vi "信号光谱9-Au-卍-ver1.vi"() -> ()   [LabVIEW 2018]
uses:
  <vilib>/Utility/NIReport.llb/Report Type.ctl
  <vilib>/Utility/file.llb/Write Delimited Spreadsheet (DBL).vi
  <vilib>/Instr/_visa.llb/VISA Configure Serial Port (Instr).vi
  <vilib>/addons/_office/excel.llb/Excel Get Data ([str]).vi
  <vilib>/Utility/NIReport.llb/NI_report.lvclass
  <vilib>/Analysis/NI_AALBase.lvlib
  <vilib>/ptbypt/NI_PtbyPt.lvlib
  <vilib>/Utility/NIReport.llb/NI_ReportGenerationCore.lvlib
  <vilib>/addons/_office/NI_ReportGenerationToolkit.lvlib
  <vilib>/Utility/NIReport.llb/Excel/NI_Excel.lvclass
panel:
  in  "num":i32=1
  in  "角度判断下限":dbl=1.0 format="%#_13g"
  in  "角度判断上限":dbl=4.0 format="%#_13g"
  out "原始峰值":dbl
  out "拟合峰值":dbl
  in  "角度倍乘系数":dbl=1.5
  out "结果展示":dbl[][](array[numeric])=[[37.33100777239877, 2672.955043835526, 29.54153292599307, 222755.0, 50.0], [37.36593979472361, 2672.656498058864, 30.113284142729572, 222833.0, 50.0], [38.96986225690859, 2673.3337152325566, 33.38805102415213, 222910.0, 75.0], [37.39946104045098, 2676.4005085744548, 31.215565446104666, 222948.0, 47.0], [35.862209164247574, 2671.7826876859012, 30.355582265151796, 223028.0, 47.0]]
  out "Δw2>C":bool=TRUE
  out "Δw1>C":bool=TRUE
  out "θi":dbl
  in  "w0":dbl format="%#_13g"
  in  "C=w-w0":dbl=180.0 format="%#_13g"
  in  "上升下降沿/s":dbl format="%.2p"
  in  "延时/s":dbl format="%.2p"
  in  "占空比/%":dbl=3.0 format="%.2p"
  in  "高电平/V":dbl=4.0 format="%.2p"
  in  "频率/Hz":dbl=6000.0 format="%.3p"
  in  "低电平/V":dbl min=0.0 max=5.0 format="%.2p"
  in  "Enable":bool
  in  "上升下降沿":i32(ring)=1 items=["上升沿", "下降沿"]
  in  "输出信号波形":u16(ring) items=["Pulse"]
  out "Output":bool
  in  "VISA 信号发生器":refnum<visa-resource-name>="USB0::0x1AB1::0x0641::DG4E192200870::INSTR"
  out "Output 2":bool
  in  "Enable 2":bool
  in  "上升下降沿/s 2":dbl format="%.2p"
  in  "延时/s 2":dbl format="%.2p"
  in  "占空比/% 2":dbl=3.0 format="%.2p"
  in  "高电平/V 2":dbl=0.002 format="%.2p"
  in  "频率/Hz 2":dbl=6000.0 format="%.3p"
  in  "低电平/V 2":dbl min=0.0 max=5.0 format="%.2p"
  in  "上升下降沿 2":i32(ring)=1 items=["上升沿", "下降沿"]
  in  "输出信号波形 2":u16(ring) items=["Pulse"]
  in  "终止测量":bool
  in  "测量次数":i32=1
  out "best fit":cluster{"Y":dbl[], "Y":dbl[]}[](graph)
  in  "拟合终点":i32=850
  in  "拟合起点":i32=200
  out "angle":dbl
  out "图片地址":string
  in  "开光时间/ms":u32=50
  out "最终存储路径 2":path
  out "照明光error out":errorcluster
  in  "照明光":bool
  in  "stop bits (10: 1 bit)":u16(ring)=10 items=["1.0"=10, "1.5"=15, "2.0"=20]
  in  "parity (0:none)":enum16{"None", "Odd", "Even", "Mark", "Space"}(ring)
  in  "data bits (8)":u16=8 min=5 max=8 step=1
  in  "baud rate":u32=9600 caption="baud rate (115200)" min=9600 max=115200
  in  "照明光VISA":refnum<visa-resource-name>="COM6"
  out "正在测量":bool
  in  "滤波阈值":dbl=3000.0 format="%#_13g"
  out "范围内？":bool[](array[boolean])
  out "w":dbl
  out "xc":dbl
  out "拟合参数":dbl[](array[numeric])
  out "最终存储路径":path
  in  "停止程序":bool
  out "configure error out":errorcluster
  in  "设置参数":bool
  out "output control error  4":errorcluster
  in  "低电平持续输出":bool
  out "output control error  5":errorcluster
  out "output control error":errorcluster
  in  "开始测量":bool
  in  "channel输出口":i32(ring) items=["Channel 1", "Channel 2"]
  out "output control error":errorcluster
  out "Spectrum":cluster{"Y":dbl[], "Y":dbl[]}[](graph)
  out "波长范围":dbl[](array[numeric])
  in  "?":enum32{"IHR 550", "CCD"}(tab)
  in  "Move To\nTarget Positions":bool
  out "Current UniqueID":string="Mono4"
  in  "Mono ID":string(combo)="Mono1"
  in  "Connect":bool
  out "Initialized JY":bool=TRUE
  in  "Force\nInitialization":bool
  in  "Target Grating":string(combo)="2"
  out "Current Description":string="1" caption="Description"
  out "Grating Index":i32=1
  out "Current Grating":dbl=1200.0
  out "Units":string="nm"
  out "Current WL":dbl=897.9988
  out "Exit Mirror\nPosition":i32(ring)=2 items=["EntranceMirror", "ExitMirror", "Front", "Side"]
  out "Entrance Mirror\nPosition":i32(ring)=2 items=["EntranceMirror", "ExitMirror", "Front", "Side"]
  out "Units 2":string="mm"
  out "Front Entrance":dbl
  in  "Target WL":dbl=516.0
  in  "Exit Mirror":u16(ring)=3 caption="Target Position Exit Mirror" items=["Front"=2, "Side"=3]
  in  "Entrance Mirror":u16(ring)=2 caption="Target Position\nEntrance Mirror" items=["Front"=2, "Side"=3]
  in  "Target\nFront Entrance":dbl=1.0
  in  "Commande tab":T1(tab)
  in  "Area Number to Display":i32
  in  "Reformat":bool
  in  "GAIN":u16(ring)=2 caption="Device Name" items=["High Light", "Best Dynamic Range", "High Sensitivity"]
  in  "ADC":u16(ring) caption="Device Name" items=["20 kHz       ", " 1 MHz       ", " 1 MHz Ultra "]
  in  "Number of Areas :":u16=1 min=1 step=1
  in  "Integration time (ms) :":i16=1000
  out "Uniques ID":u16(ring) items=["CCD1", "CCD2"]
  in  "Device Name":u16(ring) items=["Synapse CCD (Lateral)", "Synapse_IGA (Axial)"]
  in  "Signal type :":enum16{"TTL Rising Edge", "TTL Falling Edge"}(ring)=enum."TTL Falling Edge"
  in  "Trigger Type :":u16(ring) items=["On Start"=1, "Per Acquisition"=2]
  in  "trigSigTypeString":string
  in  "trigEventString":string
  in  "Enable InputTriggers :":bool
  in  "Number of Cleans":i32=1
  in  "MultiAcqShutterMode":i32(ring)=3 items=["Open For All Spectra"=1, "Open for Each Spectrum"=3]
  in  "Accumulations:":u16=10 min=1 step=1
  in  "Multi Accumulation mode:":bool
  out "Y Pixels:":i32=256
  out "DataSize":i32=1024
  out "X Pixels:":i32=1024
  out "Firmware\nVersion":string="V1.20 CCD_4000"
  out "initialized ?":bool=TRUE
  in  "Continuous":bool
  in  "CCD Busy":bool
  out "indicator":string="Ready !"
  in  "initialize":bool
  in  "ShutterOpen":bool=TRUE caption="Shutter enable"
  in  "Acquire":bool
  in  "Temperature":bool
  in  "Setup":bool
  out "Acq Time(ms)":u32=3401
  in  "Save Backlight":bool
  in  "cut backlight":bool
  out "backlight":bool=TRUE
  in  "是否拟合":bool
  in  "是否保存":bool
  in  "Close":bool=TRUE
  out "JYCCDLib.IJYCCDReqd":refnum<k7>
  out "areas :":i32[][](array[numeric])=[[1], [1], [1], [1024], [256], [1], [256]]
  in  "Constante de condition\n(Voir l'aide contextuelle)":bool
  out "temp graph":dbl(graph)=-134.538067
  out "ADC Number":i32[](array[numeric])=[0, 1, 2, 3, 4]
  out "Gain Number":i32[](array[numeric])=[10, 11, 12, 13, 8, 2]
  out "trigAddress":i32
  out "Data":i32[][](graph)
  out "error out":errorcluster
  out "Gratings":dbl[](array[numeric])=[1200.0, 300.0]
  out "Backlight":i32[][](graph)
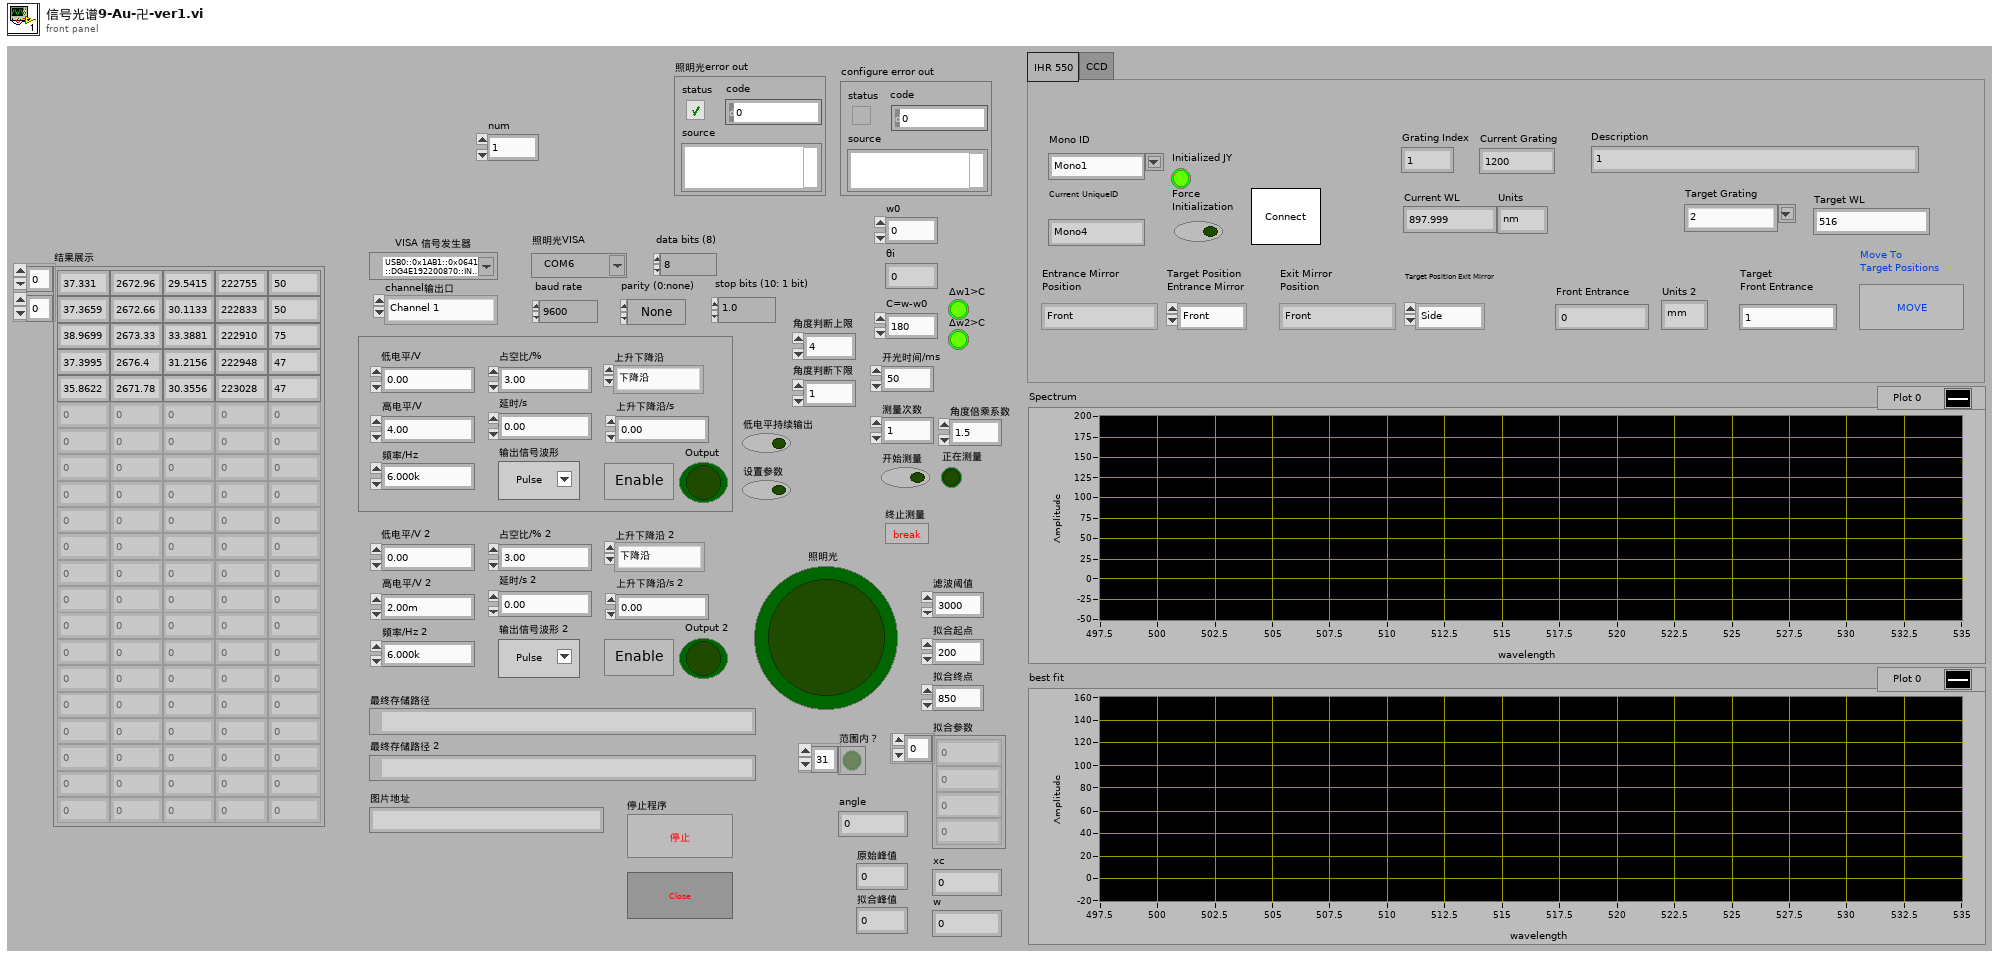
[diagram p1: front panel]
types:
  T1 = enum32{"Settings", "Trigger In", "Multi-Accu.", "Infos"}
  T2 = enum8{"Enabled", "Disabled", "Disabled and Grayed Out"}
  T3 = enum16{"maximized", "minimized", "normal", "no change"}
  T4 = typedef "NI_ReportGenerationCore.lvlib/Report Type.ctl" = enum16{"HTML", "Word", "Excel"}
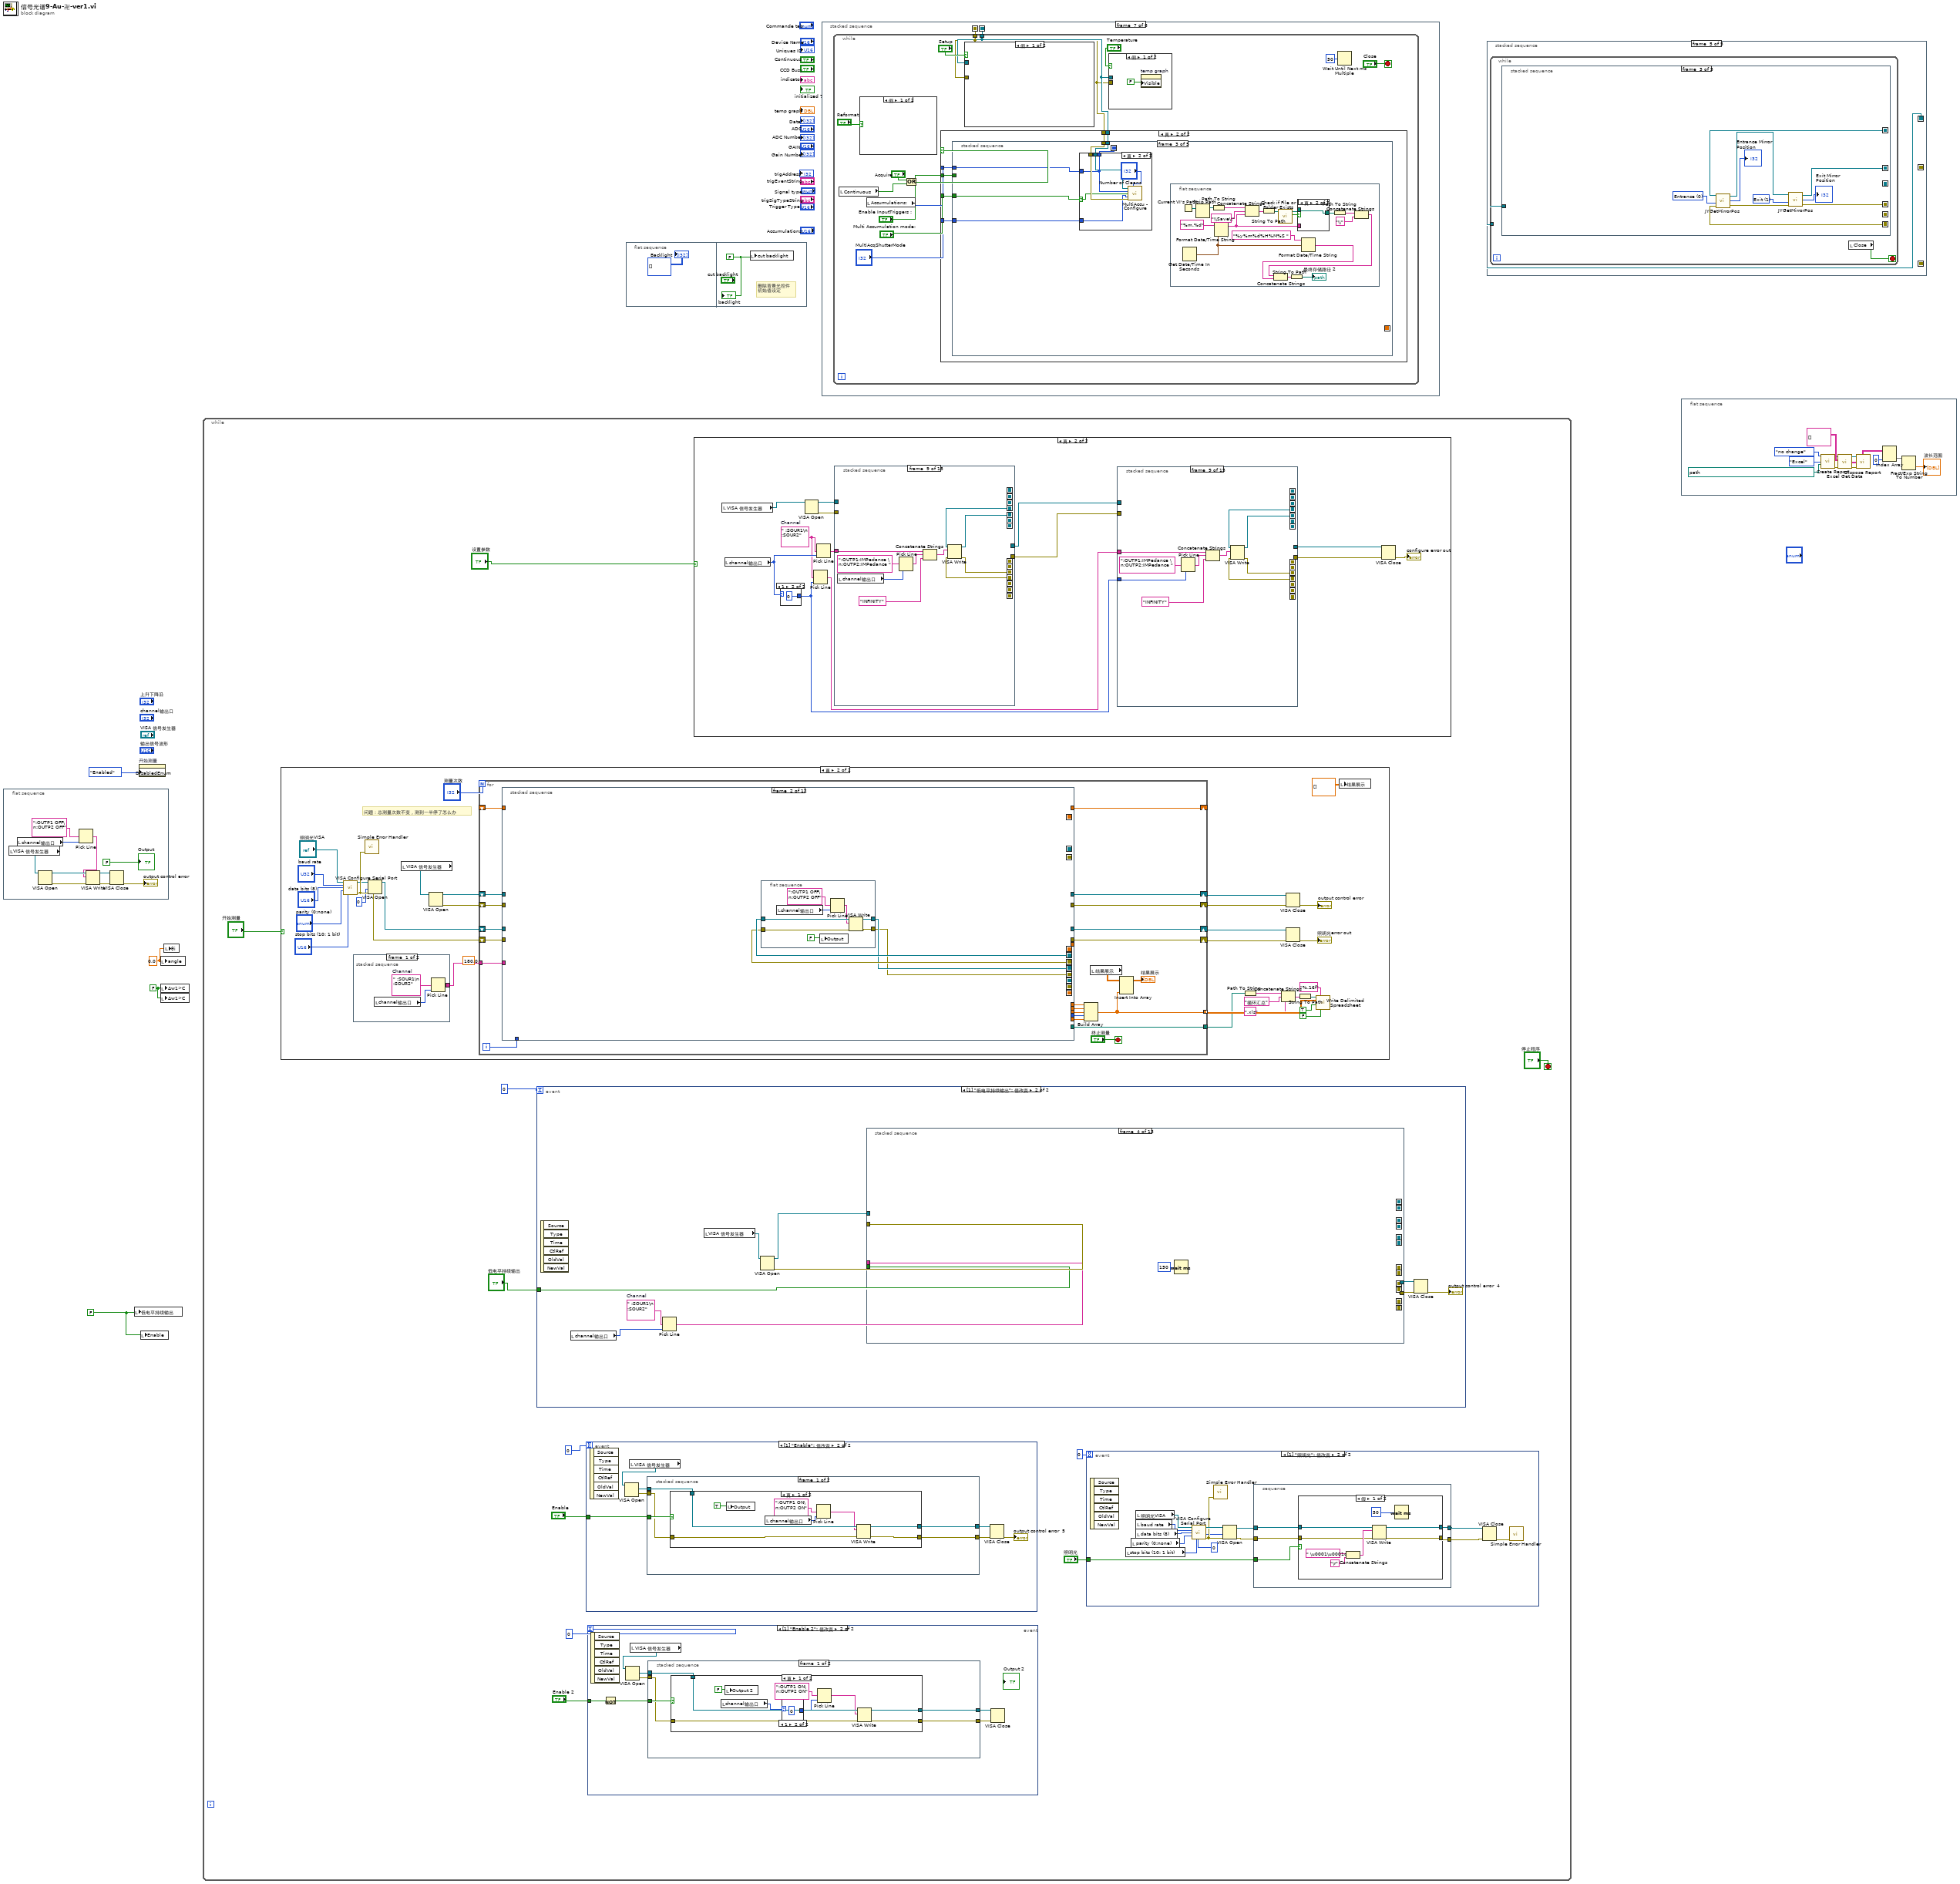
[diagram p0: block diagram]
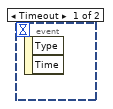
[diagram p2: hidden frame]
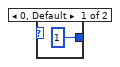
[diagram p3: hidden frame]
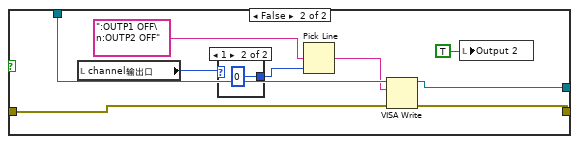
[diagram p4: hidden frame]
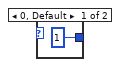
[diagram p5: hidden frame]
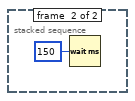
[diagram p6: hidden frame]
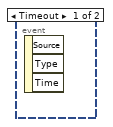
[diagram p7: hidden frame]
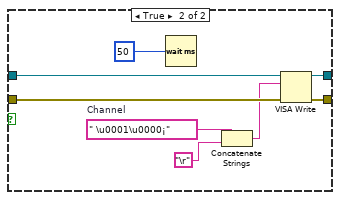
[diagram p8: hidden frame]
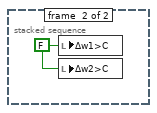
[diagram p10: hidden frame]
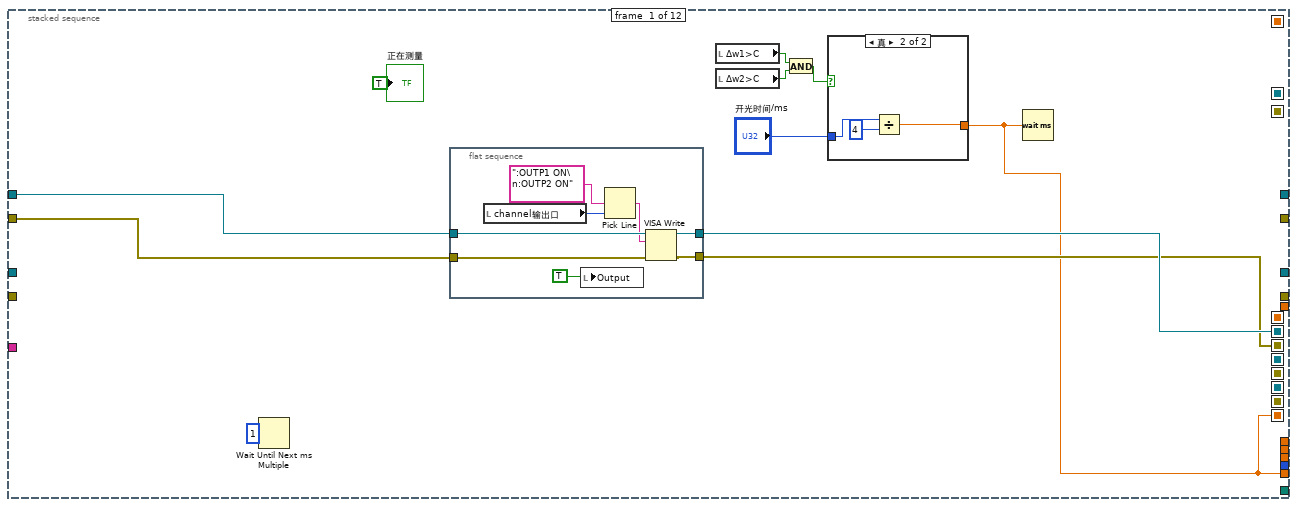
[diagram p11: hidden frame]
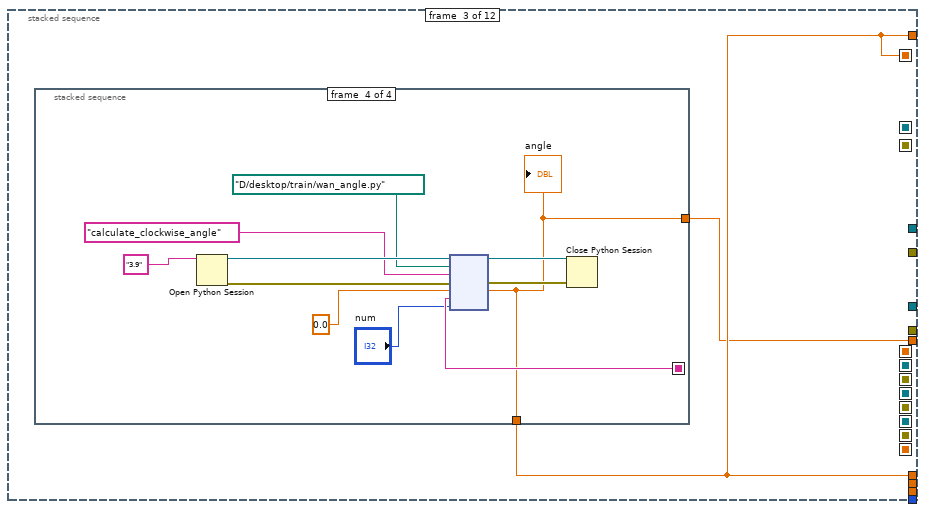
[diagram p13: hidden frame]
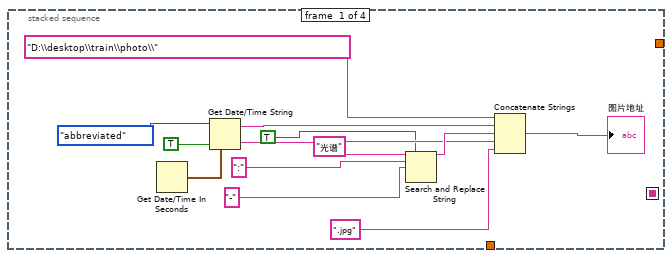
[diagram p14: hidden frame]
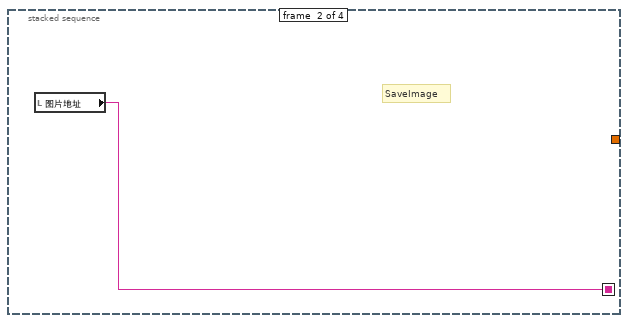
[diagram p15: hidden frame]
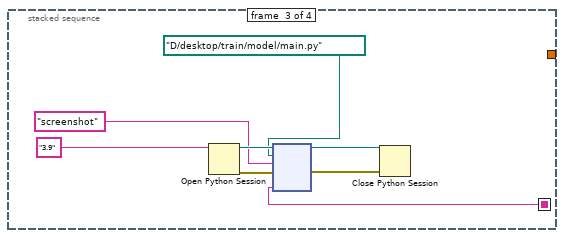
[diagram p16: hidden frame]
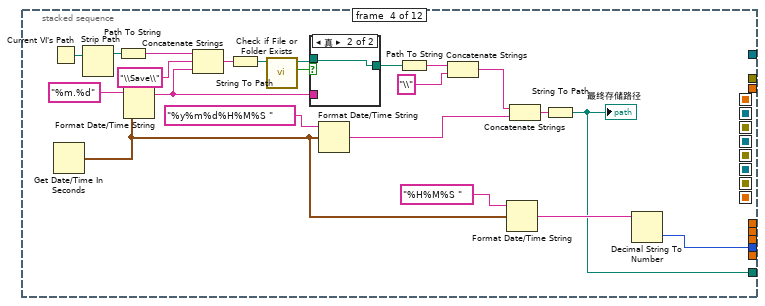
[diagram p17: hidden frame]
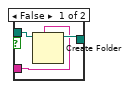
[diagram p18: hidden frame]
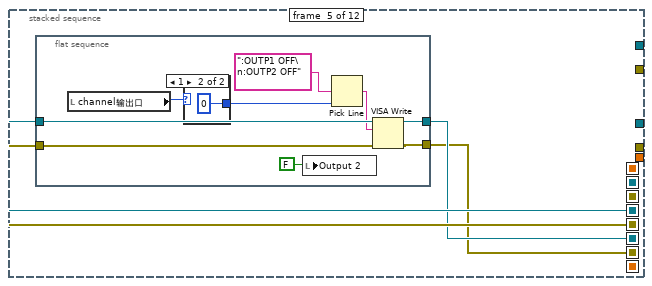
[diagram p19: hidden frame]
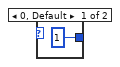
[diagram p20: hidden frame]
diagram:
  w1 = FALSE ("Δw1>C")
  w2 = 0.0 ("angle")
  w3 = FALSE
  n1 = flat-sequence {
    frame #0 {
      n2 = local read "VISA 信号发生器"() -> (w8:refnum<visa-resource-name>)
      n3 = local read "channel输出口"() -> (w6:i32)
      n4 = VISA Open(VISA resource name=w8) -> (VISA resource name=w14:refnum<visa-resource-name>, error out=w13:errorcluster)  [unwired: 4 in]
      n5 = Pick Line(multi-line string=":OUTP1 OFF\n:OUTP2 OFF" ("write buffer"), line index=w6) -> (output string=w5:string)  [unwired: 1 in]
      n6 = VISA Write(VISA resource name=w14, write buffer=w5, error in (no error)=w13) -> (VISA resource name out=w11:refnum<visa-resource-name>, error out=w10:errorcluster)  [unwired: 1 out]
      n7 = VISA Close(VISA resource name=w11, error in (no error)=w10) -> (error out=→"output control error":errorcluster)
      "Output" <- FALSE ("布尔")
    }
  }
  n8 = local write "低电平持续输出"(w3) -> ()
  n9 = property on="开始测量" class="Bool"("DisabledEnum"=T2."Enabled" ("禁用")) -> ()  [unwired: 2 in, 2 out]
  n10 = local write "Enable"(w3) -> ()
  n11 = local write "angle"(w2) -> ()
  n12 = local write "Δw1>C"(w1) -> ()
  n13 = local write "Δw1>C"(w1) -> ()
  n14 = local write "θi"(w2) -> ()
  n15 = while {
    stop <- "停止程序" stop-if-true
    n16 = case shown="真" "开始测量" {
      frame False {
      }
      frame True {
        (unwired) 180.0
        # "问题：总测量次数不变，测到一半停了怎么办"
        n17 = call-poly "VISA Configure Serial Port"("VISA resource name"="照明光VISA", "baud rate (9600)"="baud rate", "data bits (8)"="data bits (8)", "parity (0:none)"="parity (0:none)", "stop bits (10: 1 bit)"="stop bits (10: 1 bit)") -> ("VISA resource name out"=w118:refnum<visa-resource-name>, "error out"=w119:errorcluster)  [unwired: 9 in]
        n18 = stacked-sequence {
          tunnel: [w128 _] -> w122
          frame #0 {
            w129 = " :SOUR1\n :SOUR2"  # Channel
            n19 = local read "channel输出口"() -> (w130:i32)
            n20 = Pick Line(multi-line string=w129, line index=w130) -> (output string=w128:string)  [unwired: 1 in]
          }
          frame #1 {
            w131 = FALSE ("Δw1>C")
            n21 = local write "Δw1>C"(w131) -> ()
            n22 = local write "Δw2>C"(w131) -> ()
          }
        }
        n23 = call <vilib>:"Simple Error Handler.vi"("error in (no error)"=w119) -> ()  [unwired: 4 in, 5 out]
        n24 = VISA Open(access mode=0, error in (no error)=w119, VISA resource name=w118) -> (VISA resource name=w111:refnum<visa-resource-name>, error out=w110:errorcluster)  [unwired: 2 in]
        n25 = local read "VISA 信号发生器"() -> (w127:refnum<visa-resource-name>)
        n26 = VISA Open(VISA resource name=w127) -> (VISA resource name=w126:refnum<visa-resource-name>, error out=w125:errorcluster)  [unwired: 4 in]
        n27 = for {
          N: "测量次数" -> [_]
          tunnel: w122 -> [w151]
          shift-right: [w147] -> w121
          shift-left: w126 -> [w153]
          shift-right: [w146] -> w120
          shift-left: w125 -> [w152]
          shift-right: [w145] -> w124
          shift-left: w111 -> [w150]
          shift-right: [w144] -> w123
          shift-left: w110 -> [w149]
          tunnel: [w134] -> w100 mode=indexing
          shift-right: [w139] -> _
          shift-left: _ -> [w138]
          tunnel: [w135] -> w97
          i -> [w137]
          stop <- "终止测量" stop-if-true
          n28 = stacked-sequence {
            seq-local: [w160 _ _ _ _ _ _ _ _ _ _ _] -> [_ w180 _ _ _ _ _ _ _ _ _ _]
            seq-local: [w159 _ _ _ _ _ _ _ _ _ _ _] -> [_ w179 _ _ _ _ _ _ _ _ _ _]
            seq-local: [_ _ _ _ _ w267 _ _ _ _ _ _] -> [_ _ _ _ _ _ _ _ w385 _ _ _]
            seq-local: [_ _ _ _ _ w266 _ _ _ _ _ _] -> [_ _ _ _ _ _ _ _ w388 _ _ _]
            seq-local: [_ w178 _ _ _ _ _ _ _ _ _ _] -> [_ _ _ _ w253 _ _ _ _ _ _ _]
            seq-local: [_ w177 _ _ _ _ _ _ _ _ _ _] -> [_ _ _ _ w252 _ _ _ _ _ _ _]
            seq-local: [_ _ _ _ w251 _ _ _ _ _ _ _] -> [_ _ _ _ _ _ _ w371 _ _ _ _]
            seq-local: [_ _ _ _ w250 _ _ _ _ _ _ _] -> [_ _ _ _ _ _ _ w370 _ _ _ _]
            seq-local: [_ _ w190 _ _ _ _ _ _ _ _ _] -> [_ _ _ _ _ _ _ _ _ _ w397 _]
            seq-local: [_ _ _ _ _ _ w280 _ _ _ _ _] -> [_ _ _ _ _ _ _ _ _ _ w392 _]
            seq-local: [w154 _ _ _ _ _ _ _ _ _ _ _] -> [_ _ _ _ _ _ w278 _ _ _ _ _]
            tunnel: w153 -> [w162 _ _ _ _ _ _ _ _ _ _ _]
            tunnel: w152 -> [w161 _ _ _ _ _ _ _ _ _ _ _]
            tunnel: [_ _ _ _ _ _ _ w369 _ _ _ _] -> w147
            tunnel: [_ _ _ _ _ _ _ w368 _ _ _ _] -> w146
            tunnel: w151 -> [_ _ _ _ _ _ _ _ _ _ _ _]
            tunnel: w150 -> [_ _ _ _ _ w270 _ _ _ _ _ _]
            tunnel: w149 -> [_ _ _ _ _ w269 _ _ _ _ _ _]
            tunnel: [_ _ _ _ _ _ _ _ w387 _ _ _] -> w145
            tunnel: [_ _ _ _ _ _ _ _ w386 _ _ _] -> w144
            tunnel: [_ _ w190 _ _ _ _ _ _ _ _ _] -> w143
            tunnel: [_ _ _ _ _ _ w275 _ _ _ _ _] -> w142
            tunnel: [_ _ _ _ _ _ w274 _ _ _ _ _] -> w141
            tunnel: [_ _ _ w225 _ _ _ _ _ _ _ _] -> w140
            tunnel: [w154 _ _ _ _ _ _ _ _ _ _ _] -> w136
            tunnel: [_ _ w190 _ _ _ _ _ _ _ _ _] -> w139
            tunnel: w138 -> [_ _ _ _ _ _ _ _ _ _ w396 _]
            tunnel: w137 -> [_ _ _ _ _ _ _ _ _ _ w394 _]
            tunnel: [_ _ _ w224 _ _ _ _ _ _ _ _] -> w135
            tunnel: [_ _ w189 _ _ _ _ _ _ _ _ _] -> _
            frame #0 {
              n29 = Wait Until Next ms Multiple(millisecond multiple=u32 1 ("毫秒倍数")) -> ()  [unwired: 1 out]
              n30 = flat-sequence {
                tunnel: w162 -> [w176]
                tunnel: w161 -> [w175]
                tunnel: [w170] -> w160
                tunnel: [w169] -> w159
                frame #0 {
                  n31 = local read "channel输出口"() -> (w172:i32)
                  n32 = local write "Output"(TRUE ("布尔")) -> ()
                  n33 = Pick Line(multi-line string=":OUTP1 ON\n:OUTP2 ON" ("write buffer"), line index=w172) -> (output string=w171:string)  [unwired: 1 in]
                  n34 = VISA Write(VISA resource name=w176, write buffer=w171, error in (no error)=w175) -> (VISA resource name out=w170:refnum<visa-resource-name>, error out=w169:errorcluster)  [unwired: 1 out]
                }
              }
              n35 = local read "Δw1>C"() -> (w156:bool)
              n36 = local read "Δw2>C"() -> (w157:bool)
              n37 = And(x=w156, y=w157) -> (x .and. y?=w155:bool)
              n38 = case shown="真" w155 {
                tunnel: [w165 w166] -> w154
                tunnel: "开光时间/ms" -> [w165 w168]
                frame False {
                }
                frame True {
                  n39 = Divide(x=w168, y=u32 4) -> (x/y=w166:dbl)
                }
              }
              n40 = Wait (ms)(milliseconds to wait=w154) -> ()  [unwired: 1 out]
              "正在测量" <- TRUE
            }
            frame #1 {
              n41 = flat-sequence {
                tunnel: w180 -> [w188]
                tunnel: w179 -> [w187]
                tunnel: [w182] -> w178
                tunnel: [w181] -> w177
                frame #0 {
                  n42 = local read "channel输出口"() -> (w184:i32)
                  n43 = local write "Output"(FALSE ("布尔")) -> ()
                  n44 = Pick Line(multi-line string=":OUTP1 OFF\n:OUTP2 OFF" ("write buffer"), line index=w184) -> (output string=w183:string)  [unwired: 1 in]
                  n45 = VISA Write(VISA resource name=w188, write buffer=w183, error in (no error)=w187) -> (VISA resource name out=w182:refnum<visa-resource-name>, error out=w181:errorcluster)  [unwired: 1 out]
                }
              }
            }
            frame #2 {
              n46 = stacked-sequence {
                seq-local: [_ w204 _ _] -> [_ _ w205 w215]
                tunnel: [_ _ _ w213] -> w190
                tunnel: [_ _ _ w213] -> w189
                frame #0 {
                  n47 = Get Date/Time In Seconds() -> (seconds since 1Jan1904=w200:timestamp)
                  n48 = Get Date/Time String(date format (0)=enum16{"short", "long", "abbreviated"}."abbreviated" ("日期格式(0)"), seconds (now)=w200, want seconds? (F)=TRUE ("需要秒？(F)")) -> (date string=w203:string, time string=w201:string)
                  n49 = Search and Replace String(replace all?=TRUE ("替换全部？(F)"), input string=w201, search string=":" ("搜索字符串"), replace string="-" ("替换字符串(\"\")")) -> (result string=w202:string)  [unwired: 4 in, 3 out]
                  n50 = Concatenate Strings("D:\\desktop\\train\\photo\\", w203, w202, "光谱" ("字符串"), ".jpg" ("字符串")) -> (→"图片地址":string)
                }
                frame #1 {
                  # "SaveImage"
                  n51 = local read "图片地址"() -> (w204:string)
                }
                frame #2 {
                  n52 = Open Python Session(python version="3.9" ("Python version")) -> (session out=w212:refnum<k35>, error out=w210:errorcluster)  [unwired: 2 in]
                  n53 = node(w212, path "D:/desktop/train/model/main.py" ("module path"), "screenshot" ("function name"), w210, w205) -> (w211:refnum<k35>, w209:errorcluster)  [unwired: 3 in, 2 out]
                  n54 = Close Python Session(session in=w211, error in=w209) -> ()  [unwired: 1 out]
                }
                frame #3 {
                  n55 = Open Python Session(python version="3.9" ("Python version")) -> (session out=w222:refnum<k35>, error out=w220:errorcluster)  [unwired: 2 in]
                  n56 = node(w222, path "D:/desktop/train/wan_angle.py" ("module path"), "calculate_clockwise_angle" ("function name"), w220, 0.0, w215, "num") -> (w221:refnum<k35>, w219:errorcluster, w213:dbl)  [unwired: 2 in, 2 out]
                  "angle" <- w213
                  n57 = Close Python Session(session in=w221, error in=w219) -> ()  [unwired: 1 out]
                }
              }
            }
            frame #3 {
              n58 = Current VI's Path() -> (path=w234:path)
              n59 = Get Date/Time In Seconds() -> (seconds since 1Jan1904=w227:timestamp)
              n60 = Strip Path(path=w234) -> (stripped path=w235:path)  [unwired: 1 out]
              n61 = Path To String(path=w235) -> (string=w236:string)
              n62 = Format Date/Time String(time format string (%c)="%m.%d" ("时间格式字符串(%c)"), seconds (now)=w227) -> (date/time string=w242:string)  [unwired: 1 in]
              n63 = Concatenate Strings(w236, "\\Save\\" ("字符串"), w242) -> (w237:string)
              n64 = String To Path(string=w237) -> (path=w238:path)
              n65 = call <vilib>:"Check if File or Folder Exists.vi"("path"=w238) -> ("file or folder exists?"=w239:bool, "dup path"=w241:path)  [unwired: 8 in, 1 out]
              n66 = case shown="真" w239 {
                tunnel: [w248 w249] -> w240
                tunnel: w241 -> [w247 w249]
                tunnel: w242 -> [w246 _]
                frame False {
                  n67 = Create Folder(prompt (Create Folder)=w246, path (use dialog)=w247) -> (created path=w248:path)  [unwired: 1 in, 2 out]
                }
                frame True {
                }
              }
              n68 = Format Date/Time String(time format string (%c)="%y%m%d%H%M%S " ("时间格式字符串(%c)"), seconds (now)=w227) -> (date/time string=w245:string)  [unwired: 1 in]
              n69 = Path To String(path=w240) -> (string=w243:string)
              n70 = Concatenate Strings(w243, "\\" ("字符串")) -> (w244:string)
              n71 = Format Date/Time String(time format string (%c)="%H%M%S " ("时间格式字符串(%c)"), seconds (now)=w227) -> (date/time string=w226:string)  [unwired: 1 in]
              n72 = Concatenate Strings(w244, w245) -> (w233:string)
              n73 = String To Path(string=w233) -> (path=w224:path)
              "最终存储路径" <- w224
              n74 = Decimal String To Number(string=w226) -> (number=w225:i32)  [unwired: 2 in, 1 out]
            }
            frame #4 {
              n75 = flat-sequence {
                tunnel: w253 -> [w262]
                tunnel: w252 -> [w261]
                tunnel: [w257] -> w251
                tunnel: [w256] -> w250
                frame #0 {
                  n76 = local read "channel输出口"() -> (w255:i32)
                  n77 = case shown="1" w255 {
                    tunnel: [1 0] -> w254
                    frame 0, Default {
                    }
                    frame 1 {
                    }
                  }
                  n78 = local write "Output 2"(FALSE ("布尔")) -> ()
                  n79 = Pick Line(multi-line string=":OUTP1 OFF\n:OUTP2 OFF" ("write buffer"), line index=w254) -> (output string=w258:string)  [unwired: 1 in]
                  n80 = VISA Write(VISA resource name=w262, write buffer=w258, error in (no error)=w261) -> (VISA resource name out=w257:refnum<visa-resource-name>, error out=w256:errorcluster)  [unwired: 1 out]
                }
              }
            }
            frame #5 {
              w265 = " \u0001\u0001¢"  # Channel
              n81 = Wait (ms)(milliseconds to wait=1200) -> ()  [unwired: 1 out]
              n82 = Concatenate Strings(w265, "\r") -> (w271:string)
              n83 = local write "照明光"(FALSE ("照明光")) -> ()
              n84 = VISA Write(VISA resource name=w270, write buffer=w271, error in (no error)=w269) -> (VISA resource name out=w267:refnum<visa-resource-name>, error out=w266:errorcluster)  [unwired: 1 out]
            }
            frame #6 {
              n85 = local read "Area Number to Display"() -> (w321:i32)
              n86 = local read "JYCCDLib.IJYCCDReqd"() -> (w317:refnum<k7>)
              n87 = Get Date/Time In Seconds() -> (seconds since 1Jan1904=w330:timestamp)
              n88 = local read "最终存储路径"() -> (w344:path)
              n89 = Get Date/Time String(date format (0)=enum16{"short", "long", "abbreviated"}."abbreviated" ("日期格式(0)"), seconds (now)=w330, want seconds? (F)=TRUE ("需要秒？(F)")) -> (date string=w338:string, time string=w333:string)
              n90 = call "MultiAccu - Acquire spectral.vi"("error in"=errorcluster {"status"=FALSE, "code"=0, "source"=""}, "Accumulations:"=u16 1, "ShutterOpen"=TRUE, "JYCCDLib.IJYCCDReqd"=w317) -> ("Acq Time(ms)"=w323:u32, "Array Out"=w322:i32[][][])  [unwired: 1 out]
              n91 = local write "Acq Time(ms)"(w323) -> ()
              n92 = local read "cut backlight"() -> (w305:bool)
              n93 = local read "backlight"() -> (w303:bool)
              n94 = Search and Replace String(replace all?=TRUE ("替换全部？(F)"), input string=w333, search string=":" ("搜索字符串"), replace string="-" ("替换字符串(\"\")")) -> (result string=w337:string)  [unwired: 4 in, 3 out]
              n95 = Path To String(path=w344) -> (string=w327:string)
              n96 = And(x=w305, y=w303) -> (x .and. y?=w304:bool)
              n97 = call "Array reset dimension.vi"("Area Number"=w321, "Array In"=w322) -> ("Array Out"=w307:i32[][])
              n98 = Concatenate Strings(w327, w338, w337, "光谱" ("字符串"), ".xls" ("字符串")) -> (w342:string)
              n99 = case shown="真" w304 {
                tunnel: [w364 w366] -> w306
                tunnel: w307 -> [w364 w365]
                frame False {
                }
                frame True {
                  n100 = local read "Backlight"() -> (w367:i32[][])
                  n101 = Subtract(x=w365, y=w367) -> (x-y=w366:i32[][])
                }
              }
              n102 = String To Path(string=w342) -> (path=w343:path)
              n103 = local write "Data"(w307) -> ()
              n104 = local read "波长范围"() -> (w286:dbl[])
              n105 = Index Array(array=w306, index (row)=0 ("索引 (行)")) -> (element=w345:i32[])  [unwired: 1 in]
              n106 = Reverse 1D Array(array=w345) -> (reversed array=w283:i32[])
              n107 = local read "angle"() -> (w285:dbl)
              n108 = local read "拟合起点"() -> (w293:i32)
              n109 = local read "拟合终点"() -> (w295:i32)
              n110 = call <vilib>:"Median Filter.vi"("left rank"=6, "X"=w283) -> ("Filtered X"=w282:dbl[])  [unwired: 8 in, 1 out]
              n111 = Build Array(w285, w278, 0.0 ("元素")) -> (w284:dbl[])
              n112 = Subtract(x=w295, y=w293) -> (x-y=w292:i32)
              n113 = call "Convert to Dynamic Data"("Array"=w286) -> ("Dynamic Data Type"=w314:dynamicdata)  [unwired: 3 in]
              n114 = call "Convert to Dynamic Data2"("Array"=w283) -> ("Dynamic Data Type"=w313:dynamicdata)  [unwired: 3 in]
              n115 = Array Subset(array=w286, index=w293, length=w292) -> (w291:dbl[])
              n116 = call "Build XY Graph"("Y Input"=w313, "X Input"=w314) -> ("XY Graph"=→"Spectrum":cluster{"Y":dbl[], "Y":dbl[]}[])  [unwired: 8 in, 1 out]
              n117 = call "转换至动态数据4"("Array"=w291) -> ("Dynamic Data Type"=w311:dynamicdata)  [unwired: 3 in]
              n118 = In Range and Coerce(upper limit="滤波阈值", x=w282, lower limit=-100.0) -> (In Range?=w298:bool[])  [unwired: 1 out]
              "范围内？" <- w298
              n119 = Not(x=w298) -> (.not. x?=w297:bool[])
              n120 = Or Array Elements(Boolean array=w297) -> (logical OR=w300:bool)
              n121 = local read "X Pixels:"() -> (w299:i32)
              n122 = local read "波长范围"() -> (w287:dbl[])
              n123 = local read "滤波阈值"() -> (w296:dbl)
              n124 = case shown="真" w300 {
                tunnel: w299 -> [_ w351]
                tunnel: w282 -> [w347 w350]
                tunnel: [w347 w349] -> w276
                tunnel: w296 -> [_ w348]
                frame False {
                }
                frame True {
                  n125 = for {
                    N: w351 -> [_]
                    tunnel: w350 -> [w355] mode=indexing
                    tunnel: [w354] -> w349 mode=indexing
                    shift-right: [w354] -> _
                    shift-left: _ -> [w353]
                    tunnel: w348 -> [w352]
                    n126 = Greater?(x=w355, y=w352) -> (0:w357:bool)
                    n127 = Less?(x=w355, y=-100.0) -> (x < y?=w358:bool)
                    n128 = Or(x=w357, y=w358) -> (x .or. y?=w356:bool)
                    n129 = case shown="真" w356 {
                      tunnel: w355 -> [w360 _]
                      tunnel: [w360 w362] -> w354
                      tunnel: w353 -> [_ w363]
                      frame False {
                      }
                      frame True {
                        n130 = call <vilib>:"Median Filter PtByPt.vi"("rank"=5, "x"=w363) -> ("Filtered x"=w362:dbl)  [unwired: 2 in, 1 out]
                      }
                    }
                  }
                }
              }
              n131 = Array Subset(array=w276, index=w293, length=w292) -> (w294:dbl[])
              n132 = call "转换至动态数据3"("Array"=w294) -> ("Dynamic Data Type"=w312:dynamicdata)  [unwired: 3 in]
              n133 = call "曲线拟合"("Locations"=w311, "Signals"=w312) -> ("best fit"=w316:dynamicdata, "non-linear coefficients"=w315:dynamicdata)  [unwired: 5 in, 3 out]
              n134 = call "从动态数据转换"("Dynamic Data Type"=w315) -> ("Array"=w308:dbl[])  [unwired: 3 in]
              "拟合参数" <- w308
              n135 = call "从动态数据转换2"("Dynamic Data Type"=w316) -> ("Array"=w277:dbl[])  [unwired: 3 in]
              n136 = Build Array(w286, w282, w277, w308, w284) -> (w346:dbl[][])
              n137 = call-poly <vilib>:"Write Delimited Spreadsheet.vi"("file path (dialog if empty)"=w343, "format (%.3f)"="%.16f", "2D data"=w346, "append to file? (new file:F)"=TRUE ("append to file? (F)"), "transpose? (no:F)"=TRUE ("transpose? (F)")) -> ()  [unwired: 9 in, 2 out]
              n138 = Index Array(array=w308, index #1=0 ("索引"), index #2=1 ("索引")) -> (element #1=→"xc":dbl, element #2=w280:dbl)
              "w" <- w280
              n139 = Bundle("波长范围"=w287, "Filtered X"=w276) -> (w290:cluster{"波长范围 ":dbl[], "Filtered X":dbl[]})  [unwired: 1 in]
              n140 = Bundle(w291, "Array"=w277) -> (w289:cluster{dbl[], "Array":dbl[]})  [unwired: 1 in]
              n141 = Array Max & Min(array=w277) -> (max value=w274:dbl)  [unwired: 3 out]
              "拟合峰值" <- w274
              n142 = Array Max & Min(array=w276) -> (max value=w275:dbl)  [unwired: 3 out]
              "原始峰值" <- w275
              n143 = Build Array(w290, w289) -> (w288:cluster{"波长范围 ":dbl[], "Array":dbl[]}[])
              n144 = local write "best fit"(w288) -> ()
            }
            frame #7 {
              n145 = flat-sequence {
                tunnel: w371 -> [w380]
                tunnel: w370 -> [w379]
                tunnel: [w375] -> w369
                tunnel: [w374] -> w368
                frame #0 {
                  n146 = local read "channel输出口"() -> (w373:i32)
                  n147 = case shown="1" w373 {
                    tunnel: [1 0] -> w372
                    frame 0, Default {
                    }
                    frame 1 {
                    }
                  }
                  n148 = local write "Output 2"(TRUE ("布尔")) -> ()
                  n149 = Pick Line(multi-line string=":OUTP1 ON\n:OUTP2 ON" ("write buffer"), line index=w372) -> (output string=w376:string)  [unwired: 1 in]
                  n150 = VISA Write(VISA resource name=w380, write buffer=w376, error in (no error)=w379) -> (VISA resource name out=w375:refnum<visa-resource-name>, error out=w374:errorcluster)  [unwired: 1 out]
                }
              }
            }
            frame #8 {
              w383 = " \u0001\u0000¡"  # Channel
              n151 = Concatenate Strings(w383, "\r") -> (w389:string)
              n152 = VISA Write(VISA resource name=w385, write buffer=w389, error in (no error)=w388) -> (VISA resource name out=w387:refnum<visa-resource-name>, error out=w386:errorcluster)  [unwired: 1 out]
              n153 = local write "照明光"(TRUE ("照明光")) -> ()
            }
            frame #9 {
              n154 = Wait (ms)(milliseconds to wait=1200) -> ()  [unwired: 1 out]
            }
            frame #10 {
              n155 = Greater Or Equal?(x=w394, y=1) -> (x >= y?=w395:bool)
              n156 = case shown="真" w395 {
                tunnel: w397 -> [_ w403]
                tunnel: w396 -> [_ w404]
                tunnel: w392 -> [w398 w405]
                frame False {
                  n157 = local write "w0"(w398) -> ()
                }
                frame True {
                  n158 = local read "Δw1>C"() -> (w402:bool)
                  n159 = case shown="真" w402 {
                    tunnel: w405 -> [w424 w444]
                    tunnel: w404 -> [w414 _]
                    tunnel: w403 -> [w415 _]
                    frame False {
                      # "判断Δw突变位置并记录当前θ值"
                      # "根据θ变化速度改变开光时间"
                      n160 = local read "w0"() -> (w422:dbl)
                      n161 = Subtract(x=w415, y=w414) -> (x-y=w417:dbl)
                      n162 = local read "开光时间/ms"() -> (w420:u32)
                      n163 = Subtract(x=w422, y=w424) -> (x-y=w427:dbl)
                      n164 = Absolute Value(x=w417) -> (abs(x)=w419:dbl)
                      n165 = Absolute Value(x=w427) -> (abs(x)=w425:dbl)
                      n166 = Greater Or Equal?(x=w419, y="角度判断上限") -> (x >= y?=w418:bool)
                      n167 = Greater Or Equal?(x=w425, y="C=w-w0") -> (x >= y?=w423:bool)
                      n168 = case shown="真" w423 {
                        tunnel: w414 -> [_ w442]
                        frame False {
                          w440 = FALSE ("Δw1>C")
                          n169 = local write "Δw1>C"(w440) -> ()
                          n170 = local write "Δw2>C"(w440) -> ()
                        }
                        frame True {
                          "θi" <- w442
                          "Δw1>C" <- TRUE ("布尔")
                        }
                      }
                      n171 = case shown="假" w418 {
                        tunnel: w419 -> [w432 _]
                        tunnel: w420 -> [w429 w439]
                        tunnel: [w428 w437] -> w421
                        frame False {
                          n172 = Less Or Equal?(x=w432, y="角度判断下限") -> (x <= y?=w430:bool)
                          n173 = case shown="真" w430 {
                            tunnel: w429 -> [w433 w436]
                            tunnel: [w433 w435] -> w428
                            frame False {
                            }
                            frame True {
                              n174 = Multiply(x=w436, y="角度倍乘系数") -> (x*y=w435:dbl)
                            }
                          }
                        }
                        frame True {
                          n175 = Divide(x=w439, y=1.6) -> (x/y=w437:dbl)
                        }
                      }
                      n176 = local write "开光时间/ms"(w421) -> ()
                    }
                    frame True {
                      # "再次判断Δw，排除坏点影响"
                      n177 = local read "Δw2>C"() -> (w443:bool)
                      n178 = case shown="假" w443 {
                        tunnel: w444 -> [w449 _]
                        frame False {
                          n179 = local read "C=w-w0"() -> (w446:dbl)
                          n180 = local read "w0"() -> (w450:dbl)
                          n181 = Subtract(x=w450, y=w449) -> (x-y=w452:dbl)
                          n182 = Absolute Value(x=w452) -> (abs(x)=w451:dbl)
                          n183 = Add(x=w446, y=0) -> (x+y=w445:dbl)
                          n184 = Greater Or Equal?(x=w451, y=w445) -> (x >= y?=w448:bool)
                          n185 = case shown="真" w448 {
                            frame False {
                              n186 = local write "θi"(0.0 ("θi")) -> ()
                              n187 = local write "Δw1>C"(FALSE ("Δw1>C")) -> ()
                            }
                            frame True {
                              "Δw2>C" <- TRUE
                            }
                          }
                        }
                        frame True {
                        }
                      }
                    }
                  }
                  n188 = local read "Δw1>C"() -> (w400:bool)
                  n189 = local read "Δw2>C"() -> (w401:bool)
                  n190 = And(x=w400, y=w401) -> (x .and. y?=w399:bool)
                  n191 = case shown="假" w399 {
                    tunnel: w403 -> [_ w406]
                    frame False {
                    }
                    frame True {
                      # "4°后重置指示灯状态"
                      n192 = local read "θi"() -> (w410:dbl)
                      n193 = Subtract(x=w406, y=w410) -> (x-y=w411:dbl)
                      n194 = Absolute Value(x=w411) -> (abs(x)=w409:dbl)
                      n195 = Greater?(x=w409, y=4.0) -> (0:w407:bool)
                      n196 = case shown="真" w407 {
                        frame False {
                        }
                        frame True {
                          w412 = FALSE ("Δw1>C")
                          n197 = local write "Δw1>C"(w412) -> ()
                          n198 = local write "Δw2>C"(w412) -> ()
                          n199 = local write "θi"(0.0 ("θ")) -> ()
                        }
                      }
                    }
                  }
                }
              }
            }
            frame #11 {
              n200 = local write "正在测量"(FALSE) -> ()
            }
          }
          n201 = Build Array(w143, w142, w141, w140, w136) -> (w134:dbl[])
          n202 = local read "结果展示"() -> (w133:dbl[][])
          n203 = Insert Into Array(array=w133, new element=w134) -> (→"结果展示":dbl[][])  [unwired: 2 in]
        }
        n204 = Path To String(path=w97) -> (string=w106:string)
        n205 = Concatenate Strings(w106, "循环汇总" ("字符串"), ".xls" ("字符串")) -> (w105:string)
        n206 = VISA Close(VISA resource name=w121, error in (no error)=w120) -> (error out=→"output control error":errorcluster)
        n207 = VISA Close(VISA resource name=w124, error in (no error)=w123) -> (error out=→"照明光error out":errorcluster)
        n208 = String To Path(string=w105) -> (path=w104:path)
        n209 = call-poly <vilib>:"Write Delimited Spreadsheet.vi"("file path (dialog if empty)"=w104, "format (%.3f)"="%.16f", "2D data"=w100, "append to file? (new file:F)"=TRUE ("append to file? (F)"), "transpose? (no:F)"=FALSE ("transpose? (F)")) -> ()  [unwired: 9 in, 2 out]
        n210 = local write "结果展示"(dbl[][] [] ("结果展示")) -> ()
      }
    }
    n211 = event shown="[1] \"低电平持续输出\": 值改变" {
      selector: _ -> [_ _]
      dyn-events: _ -> [_ _]
      timeout: u32 0 ("Time") -> [_ _]
      tunnel: "低电平持续输出" -> [_ w486]
      event Timeout {
        n212 = event-data() -> ()  [unwired: 1 in, 2 out]
      }
      event "低电平持续输出": Value Change {
        w490 = " :SOUR1\n :SOUR2"  # Channel
        n213 = event-data() -> ()  [unwired: 1 in, 6 out]
        n214 = local read "channel输出口"() -> (w491:i32)
        n215 = Pick Line(multi-line string=w490, line index=w491) -> (output string=w489:string)  [unwired: 1 in]
        n216 = local read "VISA 信号发生器"() -> (w494:refnum<visa-resource-name>)
        n217 = VISA Open(VISA resource name=w494) -> (VISA resource name=w493:refnum<visa-resource-name>, error out=w492:errorcluster)  [unwired: 4 in]
        n218 = stacked-sequence {
          seq-local: [w500 _ _ _ _ _ _ _ _ _ _ _ _] -> [_ _ w515 _ _ _ _ _ _ _ _ _ _]
          seq-local: [w499 _ _ _ _ _ _ _ _ _ _ _ _] -> [_ _ w514 _ _ _ _ _ _ _ _ _ _]
          seq-local: [_ _ w513 _ _ _ _ _ _ _ _ _ _] -> [_ _ _ _ w518 _ _ _ _ _ _ _ _]
          seq-local: [_ _ w512 _ _ _ _ _ _ _ _ _ _] -> [_ _ _ _ w519 _ _ _ _ _ _ _ _]
          seq-local: [_ _ _ _ w527 _ _ _ _ _ _ _ _] -> [_ _ _ _ _ _ w538 _ _ _ _ _ _]
          seq-local: [_ _ _ _ w526 _ _ _ _ _ _ _ _] -> [_ _ _ _ _ _ w537 _ _ _ _ _ _]
          seq-local: [_ _ _ _ _ _ w531 _ _ _ _ _ _] -> [_ _ _ _ _ _ _ _ w541 _ _ _ _]
          seq-local: [_ _ _ _ _ _ w530 _ _ _ _ _ _] -> [_ _ _ _ _ _ _ _ w540 _ _ _ _]
          seq-local: [_ _ _ _ _ _ _ _ w544 _ _ _ _] -> [_ _ _ _ _ _ _ _ _ _ w555 _ _]
          seq-local: [_ _ _ _ _ _ _ _ w543 _ _ _ _] -> [_ _ _ _ _ _ _ _ _ _ w554 _ _]
          seq-local: [_ _ _ _ _ _ _ _ _ _ w552 _ _] -> [_ _ _ _ _ _ _ _ _ _ _ _ w569]
          seq-local: [_ _ _ _ _ _ _ _ _ _ w551 _ _] -> [_ _ _ _ _ _ _ _ _ _ _ _ w568]
          tunnel: w493 -> [w505 _ _ _ _ _ _ _ _ _ _ _ _]
          tunnel: w492 -> [w498 _ _ _ _ _ _ _ _ _ _ _ _]
          tunnel: w489 -> [w497 _ w511 _ w524 _ w535 _ w545 _ w558 _ _]
          tunnel: [_ _ _ _ _ _ _ _ _ _ _ _ w567] -> w488
          tunnel: [_ _ _ _ _ _ _ _ _ _ _ _ w565] -> w487
          tunnel: w486 -> [_ _ _ _ _ _ _ _ _ _ _ _ w566]
          frame #0 {
            w502 = " PULSe"  # Function Command
            n219 = local read "输出信号波形"() -> (w496:u16)
            n220 = Concatenate Strings(w497, ":FUNC" ("string (\"\")")) -> (w503:string)
            n221 = Pick Line(string ("")=w503, multi-line string=w502, line index=w496) -> (output string=w501:string)
            n222 = VISA Write(VISA resource name=w505, write buffer=w501, error in (no error)=w498) -> (VISA resource name out=w500:refnum<visa-resource-name>, error out=w499:errorcluster)  [unwired: 1 out]
          }
          frame #1 {
            n223 = Wait (ms)(milliseconds to wait=u32 150) -> ()  [unwired: 1 out]
          }
          frame #2 {
            n224 = Number To Fractional String(use system decimal point (T)=TRUE ("使用系统小数点(T)"), number=1.0 ("数字")) -> (F-format string=w509:string)  [unwired: 2 in]
            n225 = Concatenate Strings ("连接字符串")(w511, ":VOLTage：HIGH ", w509) -> (w508:string)
            n226 = VISA Write(VISA resource name=w515, write buffer=w508, error in (no error)=w514) -> (VISA resource name out=w513:refnum<visa-resource-name>, error out=w512:errorcluster)  [unwired: 1 out]
          }
          frame #3 {
            n227 = Wait (ms)(milliseconds to wait=u32 150) -> ()  [unwired: 1 out]
          }
          frame #4 {
            # "1 电压偏置"
            n228 = Number To Fractional String(use system decimal point (T)=TRUE ("使用系统小数点(T)"), number=0.0 ("数字")) -> (F-format string=w522:string)  [unwired: 2 in]
            n229 = Concatenate Strings(w524, ":VOLTage:LOW ", w522) -> (w523:string)
            n230 = VISA Write(VISA resource name=w518, write buffer=w523, error in (no error)=w519) -> (VISA resource name out=w527:refnum<visa-resource-name>, error out=w526:errorcluster)  [unwired: 1 out]
          }
          frame #5 {
            n231 = Wait (ms)(milliseconds to wait=u32 150) -> ()  [unwired: 1 out]
          }
          frame #6 {
            n232 = local read "channel输出口"() -> (w533:i32)
            n233 = Pick Line(multi-line string=":OUTP1:IMPedance \n:OUTP2:IMPedance " ("write buffer"), line index=w533) -> (output string=w532:string)  [unwired: 1 in]
            n234 = Concatenate Strings ("连接字符串")(w535, w532, "INFINITY") -> (w536:string)
            n235 = VISA Write(VISA resource name=w538, write buffer=w536, error in (no error)=w537) -> (VISA resource name out=w531:refnum<visa-resource-name>, error out=w530:errorcluster)  [unwired: 1 out]
          }
          frame #7 {
            n236 = Wait (ms)(milliseconds to wait=u32 150) -> ()  [unwired: 1 out]
          }
          frame #8 {
            n237 = Number To Fractional String(use system decimal point (T)=TRUE ("使用系统小数点(T)"), number=0.0 ("数字")) -> (F-format string=w548:string)  [unwired: 2 in]
            n238 = Concatenate Strings(w545, ":PULSe:DELay ", w548) -> (w546:string)
            n239 = VISA Write(VISA resource name=w541, write buffer=w546, error in (no error)=w540) -> (VISA resource name out=w544:refnum<visa-resource-name>, error out=w543:errorcluster)  [unwired: 1 out]
          }
          frame #9 {
            n240 = Wait (ms)(milliseconds to wait=u32 150) -> ()  [unwired: 1 out]
          }
          frame #10 {
            w559 = ":LEADing\n:TRAiling "  # Channel
            w563 = ":PULSe:TRANsition"  # VOLTage:Offset
            n241 = local read "上升下降沿"() -> (w560:i32)
            n242 = Pick Line(multi-line string=w559, line index=w560) -> (output string=w556:string)  [unwired: 1 in]
            n243 = Number To Fractional String(use system decimal point (T)=TRUE ("使用系统小数点(T)"), number=0.0 ("数字")) -> (F-format string=w557:string)  [unwired: 2 in]
            n244 = Concatenate Strings(w558, w563, w556, w557) -> (w561:string)
            n245 = VISA Write(VISA resource name=w555, write buffer=w561, error in (no error)=w554) -> (VISA resource name out=w552:refnum<visa-resource-name>, error out=w551:errorcluster)  [unwired: 1 out]
          }
          frame #11 {
            n246 = Wait (ms)(milliseconds to wait=u32 150) -> ()  [unwired: 1 out]
          }
          frame #12 {
            n247 = case shown="假" w566 {
              tunnel: w569 -> [w577 w578]
              tunnel: [w576 w585] -> w565
              tunnel: w568 -> [w575 w583]
              tunnel: [w574 w584] -> w567
              frame True {
                n248 = local write "Output"(TRUE ("布尔")) -> ()
                n249 = local read "channel输出口"() -> (w571:i32)
                n250 = Pick Line(multi-line string=":OUTP1 ON\n:OUTP2 ON" ("write buffer"), line index=w571) -> (output string=w570:string)  [unwired: 1 in]
                n251 = VISA Write(VISA resource name=w577, write buffer=w570, error in (no error)=w575) -> (VISA resource name out=w574:refnum<visa-resource-name>, error out=w576:errorcluster)  [unwired: 1 out]
              }
              frame False {
                n252 = local read "channel输出口"() -> (w580:i32)
                n253 = Pick Line(multi-line string=":OUTP1 OFF\n:OUTP2 OFF" ("write buffer"), line index=w580) -> (output string=w579:string)  [unwired: 1 in]
                n254 = VISA Write(VISA resource name=w578, write buffer=w579, error in (no error)=w583) -> (VISA resource name out=w584:refnum<visa-resource-name>, error out=w585:errorcluster)  [unwired: 1 out]
                n255 = local write "Output"(FALSE ("布尔")) -> ()
              }
            }
          }
        }
        n256 = VISA Close(VISA resource name=w488, error in (no error)=w487) -> (error out=→"output control error  4":errorcluster)
      }
    }
    n257 = event shown="[1] \"Enable\": 值改变" {
      selector: _ -> [_ _]
      dyn-events: _ -> [_ _]
      timeout: u32 0 ("Time") -> [_ _]
      tunnel: "Enable" -> [_ w461]
      event Timeout {
        n258 = event-data() -> ()  [unwired: 1 in, 2 out]
      }
      event "Enable": Value Change {
        n259 = event-data() -> ()  [unwired: 1 in, 6 out]
        n260 = local read "VISA 信号发生器"() -> (w457:refnum<visa-resource-name>)
        n261 = VISA Open(VISA resource name=w457) -> (VISA resource name=w460:refnum<visa-resource-name>, error out=w463:errorcluster)  [unwired: 4 in]
        n262 = stacked-sequence {
          tunnel: w461 -> [w468 _]
          tunnel: w463 -> [w467 _]
          tunnel: w460 -> [w466 _]
          tunnel: [w465 _] -> w459
          tunnel: [w464 _] -> w458
          frame #0 {
            n263 = case shown="真" w468 {
              tunnel: w466 -> [w476 w484]
              tunnel: [w475 w483] -> w464
              tunnel: w467 -> [w474 w481]
              tunnel: [w473 w482] -> w465
              frame True {
                n264 = local write "Output"(TRUE ("布尔")) -> ()
                n265 = local read "channel输出口"() -> (w470:i32)
                n266 = Pick Line(multi-line string=":OUTP1 ON\n:OUTP2 ON" ("write buffer"), line index=w470) -> (output string=w469:string)  [unwired: 1 in]
                n267 = VISA Write(VISA resource name=w476, write buffer=w469, error in (no error)=w474) -> (VISA resource name out=w473:refnum<visa-resource-name>, error out=w475:errorcluster)  [unwired: 1 out]
              }
              frame False {
                n268 = local read "channel输出口"() -> (w478:i32)
                n269 = Pick Line(multi-line string=":OUTP1 OFF\n:OUTP2 OFF" ("write buffer"), line index=w478) -> (output string=w477:string)  [unwired: 1 in]
                n270 = VISA Write(VISA resource name=w484, write buffer=w477, error in (no error)=w481) -> (VISA resource name out=w482:refnum<visa-resource-name>, error out=w483:errorcluster)  [unwired: 1 out]
                n271 = local write "Output"(FALSE ("布尔")) -> ()
              }
            }
          }
          frame #1 {
            n272 = Wait (ms)(milliseconds to wait=u32 150) -> ()  [unwired: 1 out]
          }
        }
        n273 = VISA Close(VISA resource name=w459, error in (no error)=w458) -> (error out=→"output control error  5":errorcluster)
      }
    }
    n274 = event shown="[1] \"Enable 2\": 值改变" {
      selector: _ -> [_ _]
      dyn-events: _ -> [_ _]
      timeout: u32 0 ("Time") -> [_ _]
      tunnel: "Enable 2" -> [_ w27]
      event Timeout {
        n275 = event-data() -> ()  [unwired: 1 in, 2 out]
      }
      event "Enable 2": Value Change {
        n276 = event-data() -> ()  [unwired: 1 in, 6 out]
        n277 = Not(x=w27) -> (.not. x?=w26:bool)
        n278 = local read "VISA 信号发生器"() -> (w28:refnum<visa-resource-name>)
        n279 = VISA Open(VISA resource name=w28) -> (VISA resource name=w31:refnum<visa-resource-name>, error out=w32:errorcluster)  [unwired: 4 in]
        n280 = stacked-sequence {
          tunnel: w26 -> [w37 _]
          tunnel: w32 -> [w36 _]
          tunnel: w31 -> [w35 _]
          tunnel: [w34 _] -> w30
          tunnel: [w33 _] -> w29
          frame #0 {
            n281 = case shown="真" w37 {
              tunnel: w35 -> [w46 w57]
              tunnel: [w45 w56] -> w33
              tunnel: w36 -> [w44 w54]
              tunnel: [w43 w55] -> w34
              frame True {
                n282 = local read "channel输出口"() -> (w39:i32)
                n283 = local write "Output 2"(FALSE ("布尔")) -> ()
                n284 = case shown="1" w39 {
                  tunnel: [1 0] -> w38
                  frame 0, Default {
                  }
                  frame 1 {
                  }
                }
                n285 = Pick Line(multi-line string=":OUTP1 ON\n:OUTP2 ON" ("write buffer"), line index=w38) -> (output string=w40:string)  [unwired: 1 in]
                n286 = VISA Write(VISA resource name=w46, write buffer=w40, error in (no error)=w44) -> (VISA resource name out=w43:refnum<visa-resource-name>, error out=w45:errorcluster)  [unwired: 1 out]
              }
              frame False {
                n287 = local read "channel输出口"() -> (w50:i32)
                n288 = case shown="1" w50 {
                  tunnel: [1 0] -> w49
                  frame 0, Default {
                  }
                  frame 1 {
                  }
                }
                n289 = Pick Line(multi-line string=":OUTP1 OFF\n:OUTP2 OFF" ("write buffer"), line index=w49) -> (output string=w51:string)  [unwired: 1 in]
                n290 = VISA Write(VISA resource name=w57, write buffer=w51, error in (no error)=w54) -> (VISA resource name out=w55:refnum<visa-resource-name>, error out=w56:errorcluster)  [unwired: 1 out]
                n291 = local write "Output 2"(TRUE ("布尔")) -> ()
              }
            }
          }
          frame #1 {
            n292 = Wait (ms)(milliseconds to wait=u32 150) -> ()  [unwired: 1 out]
          }
        }
        n293 = VISA Close(VISA resource name=w30, error in (no error)=w29) -> ()  [unwired: 1 out]
      }
    }
    n294 = case shown="真" "设置参数" {
      frame False {
      }
      frame True {
        w592 = " :SOUR1\n :SOUR2"  # Channel
        n295 = local read "VISA 信号发生器"() -> (w594:refnum<visa-resource-name>)
        n296 = local read "channel输出口"() -> (w593:i32)
        n297 = case shown="1" w593 {
          tunnel: [1 0] -> w586
          frame 0, Default {
          }
          frame 1 {
          }
        }
        n298 = VISA Open(VISA resource name=w594) -> (VISA resource name=w597:refnum<visa-resource-name>, error out=w598:errorcluster)  [unwired: 4 in]
        n299 = Pick Line(multi-line string=w592, line index=w586) -> (output string=w587:string)  [unwired: 1 in]
        n300 = Pick Line(multi-line string=w592, line index=w593) -> (output string=w595:string)  [unwired: 1 in]
        n301 = stacked-sequence {
          seq-local: [w694 _ _ _ _ _ _ _ _ _ _ _ _ _ _] -> [_ _ w709 _ _ _ _ _ _ _ _ _ _ _ _]
          seq-local: [w693 _ _ _ _ _ _ _ _ _ _ _ _ _ _] -> [_ _ w708 _ _ _ _ _ _ _ w747 _ _ _ _]
          seq-local: [_ _ w707 _ _ _ _ _ _ _ _ _ _ _ _] -> [_ _ _ _ w718 _ _ _ _ _ _ _ _ _ _]
          seq-local: [_ _ w706 _ _ _ _ _ _ _ _ _ _ _ _] -> [_ _ _ _ w717 _ _ _ _ _ _ _ _ _ _]
          seq-local: [_ _ _ _ w716 _ _ _ _ _ _ _ _ _ _] -> [_ _ _ _ _ _ w724 _ _ _ _ _ _ _ _]
          seq-local: [_ _ _ _ w713 _ _ _ _ _ _ _ _ _ _] -> [_ _ _ _ _ _ w723 _ _ _ _ _ _ _ _]
          seq-local: [_ _ _ _ _ _ w731 _ _ _ _ _ _ _ _] -> [_ _ _ _ _ _ _ _ w742 _ _ _ _ _ _]
          seq-local: [_ _ _ _ _ _ w730 _ _ _ _ _ _ _ _] -> [_ _ _ _ _ _ _ _ w741 _ _ _ _ _ _]
          seq-local: [_ _ _ _ _ _ _ _ w735 _ _ _ _ _ _] -> [_ _ _ _ _ _ _ _ _ _ w748 _ _ _ _]
          seq-local: [_ _ _ _ _ _ _ _ w734 _ _ _ _ _ _] -> [_ _ _ _ _ _ _ _ _ _ _ _ _ _ _]
          seq-local: [_ _ _ _ _ _ _ _ _ _ w744 _ _ _ _] -> [_ _ _ _ _ _ _ _ _ _ _ _ w758 _ _]
          seq-local: [_ _ _ _ _ _ _ _ _ _ w745 _ _ _ _] -> [_ _ _ _ _ _ _ _ _ _ _ _ w757 _ _]
          seq-local: [_ _ _ _ _ _ _ _ _ _ _ _ w756 _ _] -> [_ _ _ _ _ _ _ _ _ _ _ _ _ _ w769]
          seq-local: [_ _ _ _ _ _ _ _ _ _ _ _ w755 _ _] -> [_ _ _ _ _ _ _ _ _ _ _ _ _ _ w768]
          tunnel: w597 -> [w699 _ _ _ _ _ _ _ _ _ _ _ _ _ _]
          tunnel: w598 -> [w692 _ _ _ _ _ _ _ _ _ _ _ _ _ _]
          tunnel: w595 -> [w691 _ w705 _ w712 _ w728 _ w739 _ w749 _ w759 _ w772]
          tunnel: [_ _ _ _ _ _ _ _ _ _ _ _ _ _ w767] -> w591
          tunnel: [_ _ _ _ _ _ _ _ _ _ _ _ _ _ w766] -> w590
          frame #0 {
            w696 = " PULSe"  # Function Command
            n302 = local read "输出信号波形"() -> (w690:u16)
            n303 = Concatenate Strings(w691, ":FUNC" ("string (\"\")")) -> (w697:string)
            n304 = Pick Line(string ("")=w697, multi-line string=w696, line index=w690) -> (output string=w695:string)
            n305 = VISA Write(VISA resource name=w699, write buffer=w695, error in (no error)=w692) -> (VISA resource name out=w694:refnum<visa-resource-name>, error out=w693:errorcluster)  [unwired: 1 out]
          }
          frame #1 {
            n306 = Wait (ms)(milliseconds to wait=u32 150) -> ()  [unwired: 1 out]
          }
          frame #2 {
            n307 = Number To Fractional String(use system decimal point (T)=TRUE ("使用系统小数点(T)"), number="低电平/V") -> (F-format string=w703:string)  [unwired: 2 in]
            n308 = Concatenate Strings ("连接字符串")(w705, ":VOLTage:LOW ", w703) -> (w702:string)
            n309 = VISA Write(VISA resource name=w709, write buffer=w702, error in (no error)=w708) -> (VISA resource name out=w707:refnum<visa-resource-name>, error out=w706:errorcluster)  [unwired: 1 out]
          }
          frame #3 {
            n310 = Wait (ms)(milliseconds to wait=u32 150) -> ()  [unwired: 1 out]
          }
          frame #4 {
            # "1 频率"
            n311 = Concatenate Strings(w712, ":FREQ ") -> (w719:string)
            n312 = Format Into String ("格式化写入字符串")(initial string=w719, "频率/Hz") -> (resulting string=w720:string)  [unwired: 2 in, 1 out]
            n313 = VISA Write(VISA resource name=w718, write buffer=w720, error in (no error)=w717) -> (VISA resource name out=w716:refnum<visa-resource-name>, error out=w713:errorcluster)  [unwired: 1 out]
          }
          frame #5 {
            n314 = Wait (ms)(milliseconds to wait=u32 150) -> ()  [unwired: 1 out]
          }
          frame #6 {
            n315 = Number To Fractional String(use system decimal point (T)=TRUE ("使用系统小数点(T)"), number="高电平/V") -> (F-format string=w725:string)  [unwired: 2 in]
            n316 = Concatenate Strings(w728, ":VOLTage:HIGH ", w725) -> (w727:string)
            n317 = VISA Write(VISA resource name=w724, write buffer=w727, error in (no error)=w723) -> (VISA resource name out=w731:refnum<visa-resource-name>, error out=w730:errorcluster)  [unwired: 1 out]
          }
          frame #7 {
            n318 = Wait (ms)(milliseconds to wait=u32 150) -> ()  [unwired: 1 out]
          }
          frame #8 {
            n319 = local read "channel输出口"() -> (w737:i32)
            n320 = Pick Line(multi-line string=":OUTP1:IMPedance \n:OUTP2:IMPedance " ("write buffer"), line index=w737) -> (output string=w736:string)  [unwired: 1 in]
            n321 = Concatenate Strings ("连接字符串")(w739, w736, "INFINITY") -> (w740:string)
            n322 = VISA Write(VISA resource name=w742, write buffer=w740, error in (no error)=w741) -> (VISA resource name out=w735:refnum<visa-resource-name>, error out=w734:errorcluster)  [unwired: 1 out]
          }
          frame #9 {
            n323 = Wait (ms)(milliseconds to wait=u32 150) -> ()  [unwired: 1 out]
          }
          frame #10 {
            n324 = Number To Fractional String(use system decimal point (T)=TRUE ("使用系统小数点(T)"), number="占空比/%") -> (F-format string=w751:string)  [unwired: 2 in]
            n325 = Concatenate Strings(w749, ":PULSe:DCYCle ", w751) -> (w746:string)
            n326 = VISA Write(VISA resource name=w748, write buffer=w746, error in (no error)=w747) -> (VISA resource name out=w744:refnum<visa-resource-name>, error out=w745:errorcluster)  [unwired: 1 out]
          }
          frame #11 {
            n327 = Wait (ms)(milliseconds to wait=u32 150) -> ()  [unwired: 1 out]
          }
          frame #12 {
            n328 = Number To Fractional String(use system decimal point (T)=TRUE ("使用系统小数点(T)"), number="延时/s") -> (F-format string=w762:string)  [unwired: 2 in]
            n329 = Concatenate Strings(w759, ":PULSe:DELay ", w762) -> (w760:string)
            n330 = VISA Write(VISA resource name=w758, write buffer=w760, error in (no error)=w757) -> (VISA resource name out=w756:refnum<visa-resource-name>, error out=w755:errorcluster)  [unwired: 1 out]
          }
          frame #13 {
            n331 = Wait (ms)(milliseconds to wait=u32 150) -> ()  [unwired: 1 out]
          }
          frame #14 {
            w773 = ":LEADing\n:TRAiling "  # Channel
            w778 = ":PULSe:TRANsition"  # VOLTage:Offset
            n332 = local read "上升下降沿"() -> (w774:i32)
            n333 = Pick Line(multi-line string=w773, line index=w774) -> (output string=w770:string)  [unwired: 1 in]
            n334 = Number To Fractional String(use system decimal point (T)=TRUE ("使用系统小数点(T)"), number="上升下降沿/s") -> (F-format string=w771:string)  [unwired: 2 in]
            n335 = Concatenate Strings(w772, w778, w770, w771) -> (w775:string)
            n336 = VISA Write(VISA resource name=w769, write buffer=w775, error in (no error)=w768) -> (VISA resource name out=w767:refnum<visa-resource-name>, error out=w766:errorcluster)  [unwired: 1 out]
          }
        }
        n337 = stacked-sequence {
          seq-local: [w605 _ _ _ _ _ _ _ _ _ _ _ _ _ _] -> [_ _ w620 _ _ _ _ _ _ _ _ _ _ _ _]
          seq-local: [w604 _ _ _ _ _ _ _ _ _ _ _ _ _ _] -> [_ _ w619 _ _ _ _ _ _ _ w658 _ _ _ _]
          seq-local: [_ _ w618 _ _ _ _ _ _ _ _ _ _ _ _] -> [_ _ _ _ w629 _ _ _ _ _ _ _ _ _ _]
          seq-local: [_ _ w617 _ _ _ _ _ _ _ _ _ _ _ _] -> [_ _ _ _ w628 _ _ _ _ _ _ _ _ _ _]
          seq-local: [_ _ _ _ w627 _ _ _ _ _ _ _ _ _ _] -> [_ _ _ _ _ _ w635 _ _ _ _ _ _ _ _]
          seq-local: [_ _ _ _ w624 _ _ _ _ _ _ _ _ _ _] -> [_ _ _ _ _ _ w634 _ _ _ _ _ _ _ _]
          seq-local: [_ _ _ _ _ _ w642 _ _ _ _ _ _ _ _] -> [_ _ _ _ _ _ _ _ w653 _ _ _ _ _ _]
          seq-local: [_ _ _ _ _ _ w641 _ _ _ _ _ _ _ _] -> [_ _ _ _ _ _ _ _ w652 _ _ _ _ _ _]
          seq-local: [_ _ _ _ _ _ _ _ w647 _ _ _ _ _ _] -> [_ _ _ _ _ _ _ _ _ _ w659 _ _ _ _]
          seq-local: [_ _ _ _ _ _ _ _ w646 _ _ _ _ _ _] -> [_ _ _ _ _ _ _ _ _ _ _ _ _ _ _]
          seq-local: [_ _ _ _ _ _ _ _ _ _ w655 _ _ _ _] -> [_ _ _ _ _ _ _ _ _ _ _ _ w669 _ _]
          seq-local: [_ _ _ _ _ _ _ _ _ _ w656 _ _ _ _] -> [_ _ _ _ _ _ _ _ _ _ _ _ w668 _ _]
          seq-local: [_ _ _ _ _ _ _ _ _ _ _ _ w667 _ _] -> [_ _ _ _ _ _ _ _ _ _ _ _ _ _ w682]
          seq-local: [_ _ _ _ _ _ _ _ _ _ _ _ w666 _ _] -> [_ _ _ _ _ _ _ _ _ _ _ _ _ _ w681]
          tunnel: w591 -> [w610 _ _ _ _ _ _ _ _ _ _ _ _ _ _]
          tunnel: w590 -> [w603 _ _ _ _ _ _ _ _ _ _ _ _ _ _]
          tunnel: w587 -> [w602 _ w616 _ w623 _ w639 _ w650 _ w660 _ w670 _ w677]
          tunnel: [_ _ _ _ _ _ _ _ _ _ _ _ _ _ w680] -> w589
          tunnel: [_ _ _ _ _ _ _ _ _ _ _ _ _ _ w679] -> w588
          tunnel: w586 -> [_ _ _ _ _ _ _ _ w644 _ _ _ _ _ _]
          frame #0 {
            w607 = " PULSe"  # Function Command
            n338 = Concatenate Strings(w602, ":FUNC" ("string (\"\")")) -> (w608:string)
            n339 = Pick Line(string ("")=w608, multi-line string=w607, line index="输出信号波形 2") -> (output string=w606:string)
            n340 = VISA Write(VISA resource name=w610, write buffer=w606, error in (no error)=w603) -> (VISA resource name out=w605:refnum<visa-resource-name>, error out=w604:errorcluster)  [unwired: 1 out]
          }
          frame #1 {
            n341 = Wait (ms)(milliseconds to wait=u32 150) -> ()  [unwired: 1 out]
          }
          frame #2 {
            n342 = Number To Fractional String(use system decimal point (T)=TRUE ("使用系统小数点(T)"), number="低电平/V 2") -> (F-format string=w614:string)  [unwired: 2 in]
            n343 = Concatenate Strings ("连接字符串")(w616, ":VOLTage:LOW ", w614) -> (w613:string)
            n344 = VISA Write(VISA resource name=w620, write buffer=w613, error in (no error)=w619) -> (VISA resource name out=w618:refnum<visa-resource-name>, error out=w617:errorcluster)  [unwired: 1 out]
          }
          frame #3 {
            n345 = Wait (ms)(milliseconds to wait=u32 150) -> ()  [unwired: 1 out]
          }
          frame #4 {
            # "1 频率"
            n346 = Concatenate Strings(w623, ":FREQ ") -> (w630:string)
            n347 = Format Into String ("格式化写入字符串")(initial string=w630, "频率/Hz 2") -> (resulting string=w631:string)  [unwired: 2 in, 1 out]
            n348 = VISA Write(VISA resource name=w629, write buffer=w631, error in (no error)=w628) -> (VISA resource name out=w627:refnum<visa-resource-name>, error out=w624:errorcluster)  [unwired: 1 out]
          }
          frame #5 {
            n349 = Wait (ms)(milliseconds to wait=u32 150) -> ()  [unwired: 1 out]
          }
          frame #6 {
            n350 = Number To Fractional String(use system decimal point (T)=TRUE ("使用系统小数点(T)"), number="高电平/V 2") -> (F-format string=w636:string)  [unwired: 2 in]
            n351 = Concatenate Strings(w639, ":VOLTage:HIGH ", w636) -> (w638:string)
            n352 = VISA Write(VISA resource name=w635, write buffer=w638, error in (no error)=w634) -> (VISA resource name out=w642:refnum<visa-resource-name>, error out=w641:errorcluster)  [unwired: 1 out]
          }
          frame #7 {
            n353 = Wait (ms)(milliseconds to wait=u32 150) -> ()  [unwired: 1 out]
          }
          frame #8 {
            n354 = Pick Line(multi-line string=":OUTP1:IMPedance \n:OUTP2:IMPedance " ("write buffer"), line index=w644) -> (output string=w648:string)  [unwired: 1 in]
            n355 = Concatenate Strings ("连接字符串")(w650, w648, "INFINITY") -> (w651:string)
            n356 = VISA Write(VISA resource name=w653, write buffer=w651, error in (no error)=w652) -> (VISA resource name out=w647:refnum<visa-resource-name>, error out=w646:errorcluster)  [unwired: 1 out]
          }
          frame #9 {
            n357 = Wait (ms)(milliseconds to wait=u32 150) -> ()  [unwired: 1 out]
          }
          frame #10 {
            n358 = Number To Fractional String(use system decimal point (T)=TRUE ("使用系统小数点(T)"), number="占空比/% 2") -> (F-format string=w662:string)  [unwired: 2 in]
            n359 = Concatenate Strings(w660, ":PULSe:DCYCle ", w662) -> (w657:string)
            n360 = VISA Write(VISA resource name=w659, write buffer=w657, error in (no error)=w658) -> (VISA resource name out=w655:refnum<visa-resource-name>, error out=w656:errorcluster)  [unwired: 1 out]
          }
          frame #11 {
            n361 = Wait (ms)(milliseconds to wait=u32 150) -> ()  [unwired: 1 out]
          }
          frame #12 {
            n362 = Number To Fractional String(use system decimal point (T)=TRUE ("使用系统小数点(T)"), number="延时/s 2") -> (F-format string=w673:string)  [unwired: 2 in]
            n363 = Concatenate Strings(w670, ":PULSe:DELay ", w673) -> (w671:string)
            n364 = VISA Write(VISA resource name=w669, write buffer=w671, error in (no error)=w668) -> (VISA resource name out=w667:refnum<visa-resource-name>, error out=w666:errorcluster)  [unwired: 1 out]
          }
          frame #13 {
            n365 = Wait (ms)(milliseconds to wait=u32 150) -> ()  [unwired: 1 out]
          }
          frame #14 {
            w685 = ":LEADing\n:TRAiling "  # Channel
            w689 = ":PULSe:TRANsition"  # VOLTage:Offset
            n366 = Pick Line(multi-line string=w685, line index="上升下降沿 2") -> (output string=w683:string)  [unwired: 1 in]
            n367 = Number To Fractional String(use system decimal point (T)=TRUE ("使用系统小数点(T)"), number="上升下降沿/s 2") -> (F-format string=w684:string)  [unwired: 2 in]
            n368 = Concatenate Strings(w677, w689, w683, w684) -> (w686:string)
            n369 = VISA Write(VISA resource name=w682, write buffer=w686, error in (no error)=w681) -> (VISA resource name out=w680:refnum<visa-resource-name>, error out=w679:errorcluster)  [unwired: 1 out]
          }
        }
        n370 = VISA Close(VISA resource name=w589, error in (no error)=w588) -> (error out=→"configure error out":errorcluster)
      }
    }
    n371 = event shown="[1] \"照明光\": 值改变" {
      selector: _ -> [_ _]
      dyn-events: _ -> [_ _]
      timeout: 0 -> [_ _]
      tunnel: "照明光" -> [_ w61]
      event Timeout {
        n372 = event-data() -> ()  [unwired: 1 in, 3 out]
      }
      event "照明光": Value Change {
        n373 = event-data() -> ()  [unwired: 1 in, 6 out]
        n374 = local read "stop bits (10: 1 bit)"() -> (w74:u16)
        n375 = local read "parity (0:none)"() -> (w73:enum16{"None", "Odd", "Even", "Mark", "Space"})
        n376 = local read "照明光VISA"() -> (w70:refnum<visa-resource-name>)
        n377 = local read "baud rate"() -> (w71:u32)
        n378 = local read "data bits (8)"() -> (w72:u16)
        n379 = call-poly "VISA Configure Serial Port"("VISA resource name"=w70, "baud rate (9600)"=w71, "data bits (8)"=w72, "parity (0:none)"=w73, "stop bits (10: 1 bit)"=w74) -> ("VISA resource name out"=w67:refnum<visa-resource-name>, "error out"=w66:errorcluster)  [unwired: 9 in]
        n380 = call <vilib>:"Simple Error Handler.vi"("error in (no error)"=w66) -> ()  [unwired: 4 in, 5 out]
        n381 = VISA Open(access mode=0, error in (no error)=w66, VISA resource name=w67) -> (VISA resource name=w69:refnum<visa-resource-name>, error out=w68:errorcluster)  [unwired: 2 in]
        n382 = stacked-sequence {
          tunnel: w69 -> [w79]
          tunnel: w68 -> [w78]
          tunnel: [w77] -> w64
          tunnel: [w76] -> w65
          tunnel: w61 -> [w75]
          frame #0 {
            n383 = case shown="假" w75 {
              tunnel: w79 -> [w85 w95]
              tunnel: [w83 w94] -> w77
              tunnel: w78 -> [w84 w93]
              tunnel: [w82 w92] -> w76
              frame False {
                n384 = Concatenate Strings(" \u0001\u0001¢", "\r") -> (w86:string)
                n385 = VISA Write(VISA resource name=w85, write buffer=w86, error in (no error)=w84) -> (VISA resource name out=w83:refnum<visa-resource-name>, error out=w82:errorcluster)  [unwired: 1 out]
                n386 = Wait (ms)(milliseconds to wait=50) -> ()  [unwired: 1 out]
              }
              frame True {
                w88 = " \u0001\u0000¡"  # Channel
                n387 = Wait (ms)(milliseconds to wait=50) -> ()  [unwired: 1 out]
                n388 = Concatenate Strings(w88, "\r") -> (w89:string)
                n389 = VISA Write(VISA resource name=w95, write buffer=w89, error in (no error)=w93) -> (VISA resource name out=w94:refnum<visa-resource-name>, error out=w92:errorcluster)  [unwired: 1 out]
              }
            }
          }
        }
        n390 = VISA Close(VISA resource name=w64, error in (no error)=w65) -> (error out=w63:errorcluster)
        n391 = call <vilib>:"Simple Error Handler.vi"("error in (no error)"=w63) -> ()  [unwired: 4 in, 5 out]
      }
    }
  }
  n392 = flat-sequence {
    frame #0 {
      "Backlight" <- i32[][] [] ("Backlight")
    }
    frame #1 {
      w780 = FALSE
      # "删除背景光控件\n初始值设定"
      n393 = local write "cut backlight"(w780) -> ()
      "backlight" <- w780
    }
  }
  n394 = stacked-sequence {
    seq-local: [_ _ _ w801 _ _ _ _] -> [_ _ _ _ w819 w839 w842 w1044]
    seq-local: [_ _ _ w800 _ _ _ _] -> [_ _ _ _ w820 w840 w841 w1045]
    frame #0 {
      # "initialize all variables"
      n395 = property on="initialize" class="Bool"("Désactivé"=u8 0) -> ()  [unwired: 2 in, 2 out]
      n396 = property on="Acquire" class="Bool"("Visible"=FALSE) -> ()  [unwired: 2 in, 2 out]
      n397 = property on="Setup" class="Bool"("Visible"=FALSE) -> ()  [unwired: 2 in, 2 out]
      n398 = local write "indicator"("" ("indicator")) -> ()
      n399 = local write "initialized ?"(FALSE ("initialized ?")) -> ()
      n400 = local write "Continuous"(FALSE ("Continuous")) -> ()
      n401 = local write "Close"(FALSE ("Close")) -> ()
      n402 = property on="Device Name" class="Ring (严格)"("Désactivé"=u8 0) -> ()  [unwired: 2 in, 2 out]
      n403 = property on="Continuous" class="Bool (严格)"("Visible"=FALSE) -> ()  [unwired: 2 in, 2 out]
      n404 = local write "Commande tab"(T1."Settings" ("Commande tab")) -> ()
    }
    frame #1 {
      # "Read Uniq ID"
      n405 = stacked-sequence {
        frame #0 {
          n406 = call "read detector uniq-id.vi"() -> ("nbr of components"=w793:i32, "UniqueID"=w792:string[], "Name"=w791:string[])  [unwired: 4 out]
          n407 = for {
            N: w793 -> [_]
            tunnel: w792 -> [w795]
            tunnel: w791 -> [w794]
            n408 = property on="Device Name" class="Ring (严格)"("Chaînes []"=w794) -> ()  [unwired: 2 in, 2 out]
            n409 = property on="Uniques ID" class="Ring (严格)"("Chaînes []"=w795) -> ()  [unwired: 2 in, 2 out]
          }
        }
      }
    }
    frame #2 {
      n410 = while {
        stop <- "initialize" stop-if-true
        n411 = local read "Device Name"() -> (w798:u16)
        n412 = local write "Uniques ID"(w798) -> ()
        n413 = local read "Close"() -> (w796:bool)
        n414 = Stop(stop? (T)=w796) -> ()
        n415 = Wait Until Next ms Multiple(millisecond multiple=u32 100 ("n millisecondes")) -> ()  [unwired: 1 out]
      }
    }
    frame #3 {
      n416 = stacked-sequence {
        tunnel: [_ w808 _ _] -> w801
        tunnel: [_ w807 _ _] -> w800
        frame #0 {
          n417 = local write "indicator"("Initializing ..." ("indicator")) -> ()
        }
        frame #1 {
          n418 = local read "Uniques ID"() -> (w805:u16)
          n419 = property on="Uniques ID" class="Ring (严格)"() -> ("Chaînes []"=w806:string[])  [unwired: 2 in, 2 out]
          n420 = Index Array(array=w806, index=w805) -> (element=w804:string)
          n421 = call "Initialize CCD.vi"("Unique id:"=w804) -> ("activeYPixels"=→"Y Pixels:":i32, "JYCCDLib.IJYCCDReqd"=w807:refnum<k7>, "activeXPixels"=→"X Pixels:":i32, "sortie d'erreur"=w808:errorcluster, "FirmwareVersion"=→"Firmware\nVersion":string)  [unwired: 3 out]
        }
        frame #2 {
          n422 = property on="initialize" class="Bool"("Désactivé"=u8 2) -> ()  [unwired: 2 in, 2 out]
          n423 = property on="Device Name" class="Ring (严格)"("Désactivé"=u8 2) -> ()  [unwired: 2 in, 2 out]
          n424 = local write "Continuous"(FALSE ("Continuous")) -> ()
          n425 = property on="Setup" class="Bool"("Visible"=TRUE) -> ()  [unwired: 2 in, 2 out]
        }
        frame #3 {
          n426 = local write "initialized ?"(TRUE ("initialized ?")) -> ()
          n427 = local write "indicator"("Initialized !" ("indicator")) -> ()
        }
      }
    }
    frame #4 {
      # "Actually not working"
      # "Read ADC and GAIN"
      n428 = case shown="真" "Constante de condition\n(Voir l'aide contextuelle)" {
        tunnel: w820 -> [_ w830]
        tunnel: w819 -> [_ w829]
        frame False {
        }
        frame True {
          # "Read Input supported trigger"
          n429 = call "Trigger - Get Supported Input.vi"("JYCCDLib.IJYCCDReqd"=w830, "Error Input"=w829) -> ("trigAddress"=w824:i32, "eventPtr"=w825:i32, "trigEventString"=w828:string, "trigSigType"=w827:i32, "trigSigTypeString"=w826:string)  [unwired: 4 out]
          n430 = local write "trigSigTypeString"(w826) -> ()
          n431 = local write "trigAddress"(w824) -> ()
          n432 = local write "Trigger Type :"(w825) -> ()
          n433 = local write "trigEventString"(w828) -> ()
          n434 = local write "Signal type :"(w827) -> ()
        }
      }
      n435 = call "Init ADC & Gain.vi"("JYCCDLib.IJYCCDReqd"=w820, "input error"=w819) -> ("ADC Number"=w818:i32[], "ADC description"=w823:string[], "Gain Number"=w821:i32[], "Gain description"=w822:string[])
      n436 = local write "Gain Number"(w821) -> ()
      n437 = local write "ADC Number"(w818) -> ()
      n438 = stacked-sequence {
        tunnel: w823 -> [w831 _]
        tunnel: w822 -> [_ w832]
        frame #0 {
          n439 = property on="ADC" class="Ring (严格)"("Chaînes []"=w831) -> ()  [unwired: 2 in, 2 out]
        }
        frame #1 {
          n440 = property on="GAIN" class="Ring (严格)"("Chaînes []"=w832) -> ()  [unwired: 2 in, 2 out]
        }
      }
    }
    frame #5 {
      # "IS multi Accumulation Supported ?"
      n441 = call "MultiAccu - Is Supported.vi"("Error In"=w839, "JYCCDLib.IJYCCDReqd"=w840) -> ("IsOperatingModeSupported"=w833:bool)  [unwired: 3 out]
      n442 = Select(t=0, s=w833, f=2) -> (s? t:f=w836:i32)
      n443 = Select(t=FALSE, s=w833, f=w833) -> (s? t:f=w835:bool)
      n444 = local write "Multi Accumulation mode:"(w835) -> ()
      n445 = property on="Multi Accumulation mode:" class="Bool (严格)"("Désactivé"=w836) -> ()  [unwired: 2 in, 2 out]
      n446 = property on="Multi Accumulation mode:" class="Bool (严格)"("Désactivé"=w836) -> ()  [unwired: 2 in, 2 out]
    }
    frame #6 {
      n447 = while {
        tunnel: w841 -> [w849]
        tunnel: w842 -> [w848]
        stop <- "Close" stop-if-true
        n448 = local read "Continuous"() -> (w850:bool)
        n449 = case shown="假" "Reformat" {
          frame False {
          }
          frame True {
            n450 = local read "Y Pixels:"() -> (w1022:i32)
            n451 = local read "X Pixels:"() -> (w1024:i32)
            n452 = call "Spectral Reformat CCD area.vi"("Y Pixels:"=w1022, "X Pixels:"=w1024, "numAreas"="Number of Areas :") -> ("areas :"=→"areas :":i32[][])  [unwired: 3 out]
          }
        }
        n453 = local read "Accumulations:"() -> (w845:u16)
        n454 = Or(x="Acquire", y=w850) -> (x .or. y?=w847:bool)
        n455 = case shown="真" w847 {
          tunnel: w849 -> [_ w862]
          tunnel: w848 -> [_ w861]
          tunnel: "Enable InputTriggers :" -> [_ w860]
          tunnel: "Multi Accumulation mode:" -> [_ w859]
          tunnel: w845 -> [_ w858]
          tunnel: "MultiAcqShutterMode" -> [_ w857]
          frame False {
          }
          frame True {
            n456 = stacked-sequence {
              seq-local: [_ _ w875 _ _] -> [_ _ _ w948 _]
              seq-local: [_ _ _ w921 _] -> [_ _ _ _ w988]
              tunnel: w862 -> [_ w864 w879 w947 _]
              tunnel: w861 -> [_ w865 w878 w946 _]
              tunnel: w860 -> [_ w866 _ _ _]
              tunnel: w859 -> [_ _ w877 _ _]
              tunnel: w858 -> [_ _ w876 _ _]
              tunnel: w857 -> [_ _ w874 _ _]
              frame #0 {
                n457 = local write "CCD Busy"(TRUE ("CCD Busy")) -> ()
              }
              frame #1 {
                n458 = case shown="真" w866 {
                  tunnel: w865 -> [w867 w873]
                  tunnel: w864 -> [w868 w872]
                  frame False {
                    n459 = call "Trigger - Disable.vi"("Error In"=w867, "JYCCDLib.IJYCCDReqd"=w868) -> ()  [unwired: 6 out]
                  }
                  frame True {
                    n460 = local read "Trigger Type :"() -> (w869:u16)
                    n461 = local read "Signal type :"() -> (w870:enum16{"TTL Rising Edge", "TTL Falling Edge"})
                    n462 = local read "trigAddress"() -> (w871:i32)
                    n463 = call "Trigger - Enable.vi"("Error In"=w873, "sigType"=w870, "event"=w869, "trigAddress"=w871, "JYCCDLib.IJYCCDReqd"=w872) -> ()  [unwired: 3 out]
                  }
                }
              }
              frame #2 {
                n464 = case shown="真" w877 {
                  selector: w877 -> [_ w908]
                  tunnel: w879 -> [w905 w911]
                  tunnel: w878 -> [w904 w910]
                  tunnel: w876 -> [_ w909]
                  tunnel: [u16 1 ("Accumulations:") w909] -> w875
                  tunnel: w874 -> [_ w907]
                  frame False {
                    n465 = call "MultiAccu - Disable.vi"("Error In"=w904, "JYCCDLib.IJYCCDReqd"=w905) -> ()  [unwired: 4 out]
                  }
                  frame True {
                    n466 = call "MultiAccu - Configure.vi"("JYCCDLib.IJYCCDReqd"=w911, "Cleans Before"="Number of Cleans", "Accumulations:"=w909, "MultiAcqHardwareMode"=w908, "MultiAcqShutterMode"=w907, "Error In"=w910) -> ()  [unwired: 1 in, 9 out]
                  }
                }
                n467 = flat-sequence {
                  frame #0 {
                    n468 = Current VI's Path() -> (path=w885:path)
                    n469 = Get Date/Time In Seconds() -> (seconds since 1Jan1904=w887:timestamp)
                    n470 = Strip Path(path=w885) -> (stripped path=w886:path)  [unwired: 1 out]
                    n471 = Path To String(path=w886) -> (string=w888:string)
                    n472 = Format Date/Time String(time format string (%c)="%m.%d" ("时间格式字符串(%c)"), seconds (now)=w887) -> (date/time string=w894:string)  [unwired: 1 in]
                    n473 = Concatenate Strings(w888, "\\Save\\" ("字符串"), w894) -> (w889:string)
                    n474 = String To Path(string=w889) -> (path=w890:path)
                    n475 = call <vilib>:"Check if File or Folder Exists.vi"("path"=w890) -> ("file or folder exists?"=w891:bool, "dup path"=w893:path)  [unwired: 8 in, 1 out]
                    n476 = case shown="真" w891 {
                      tunnel: [w901 w902] -> w892
                      tunnel: w893 -> [w900 w902]
                      tunnel: w894 -> [w899 _]
                      frame False {
                        n477 = Create Folder(prompt (Create Folder)=w899, path (use dialog)=w900) -> (created path=w901:path)  [unwired: 1 in, 2 out]
                      }
                      frame True {
                      }
                    }
                    n478 = Format Date/Time String(time format string (%c)="%y%m%d%H%M%S " ("时间格式字符串(%c)"), seconds (now)=w887) -> (date/time string=w897:string)  [unwired: 1 in]
                    n479 = Path To String(path=w892) -> (string=w895:string)
                    n480 = Concatenate Strings(w895, "\\" ("字符串")) -> (w896:string)
                    n481 = Concatenate Strings(w896, w897) -> (w884:string)
                    n482 = String To Path(string=w884) -> (path=→"最终存储路径 2":path)
                  }
                }
              }
              frame #3 {
                n483 = local read "cut backlight"() -> (w935:bool)
                n484 = local read "backlight"() -> (w934:bool)
                n485 = call "MultiAccu - Acquire spectral.vi"("error in"=w946, "Accumulations:"=w948, "ShutterOpen"="ShutterOpen", "JYCCDLib.IJYCCDReqd"=w947) -> ("Acq Time(ms)"=→"Acq Time(ms)":u32, "Array Out"=w945:i32[][][])  [unwired: 1 out]
                n486 = And(x=w935, y=w934) -> (x .and. y?=w936:bool)
                n487 = call "Array reset dimension.vi"("Area Number"="Area Number to Display", "Array In"=w945) -> ("Array Out"=w937:i32[][])
                n488 = case shown="真" w936 {
                  tunnel: [w984 w985] -> w938
                  tunnel: w937 -> [w984 w986]
                  frame False {
                  }
                  frame True {
                    n489 = local read "Backlight"() -> (w987:i32[][])
                    n490 = Subtract(x=w986, y=w987) -> (x-y=w985:i32[][])
                  }
                }
                n491 = local read "波长范围"() -> (w913:dbl[])
                n492 = local write "Data"(w937) -> ()
                n493 = Index Array(array=w938, index (row)=0 ("禁用的索引 (列)")) -> (element=w939:i32[])  [unwired: 1 in]
                n494 = Reverse 1D Array(array=w939) -> (reversed array=w922:i32[])
                n495 = call "转换至动态数据2"("Array"=w913) -> ("Dynamic Data Type"=w941:dynamicdata)  [unwired: 3 in]
                n496 = call "转换至动态数据"("Array"=w922) -> ("Dynamic Data Type"=w942:dynamicdata)  [unwired: 3 in]
                n497 = call <vilib>:"Median Filter.vi"("left rank"=6, "X"=w922) -> ("Filtered X"=w927:dbl[])  [unwired: 8 in, 1 out]
                n498 = call "Build XY Graph2"("Y Input"=w942, "X Input"=w941) -> ("XY Graph"=w940:cluster{"Y":dbl[], "Y":dbl[]}[])  [unwired: 8 in, 1 out]
                n499 = Subtract(x="拟合终点", y="拟合起点") -> (x-y=w916:i32)
                n500 = local write "Spectrum"(w940) -> ()
                n501 = local read "滤波阈值"() -> (w931:dbl)
                n502 = Array Subset(array=w913, index="拟合起点", length=w916) -> (w919:dbl[])
                n503 = local read "拟合参数"() -> (w912:dbl[])
                n504 = In Range and Coerce(upper limit=w931, x=w927, lower limit=-100.0) -> (In Range?=w930:bool[])  [unwired: 1 out]
                n505 = Not(x=w930) -> (.not. x?=w924:bool[])
                n506 = local read "滤波阈值"() -> (w926:dbl)
                n507 = local write "范围内？"(w930) -> ()
                n508 = local read "X Pixels:"() -> (w928:i32)
                n509 = Or Array Elements(Boolean array=w924) -> (logical OR=w929:bool)
                n510 = case shown="真" w929 {
                  tunnel: w928 -> [_ w971]
                  tunnel: w927 -> [w967 w970]
                  tunnel: [w967 w969] -> w915
                  tunnel: w926 -> [_ w968]
                  frame False {
                  }
                  frame True {
                    n511 = for {
                      N: w971 -> [_]
                      tunnel: w970 -> [w975] mode=indexing
                      tunnel: [w974] -> w969 mode=indexing
                      shift-right: [w974] -> _
                      shift-left: _ -> [w973]
                      tunnel: w968 -> [w972]
                      n512 = Greater?(x=w975, y=w972) -> (0:w977:bool)
                      n513 = Less?(x=w975, y=-100.0) -> (x < y?=w978:bool)
                      n514 = Or(x=w977, y=w978) -> (x .or. y?=w976:bool)
                      n515 = case shown="真" w976 {
                        tunnel: w975 -> [w980 _]
                        tunnel: [w980 w982] -> w974
                        tunnel: w973 -> [_ w983]
                        frame False {
                        }
                        frame True {
                          n516 = call <vilib>:"Median Filter PtByPt.vi"("rank"=5, "x"=w983) -> ("Filtered x"=w982:dbl)  [unwired: 2 in, 1 out]
                        }
                      }
                    }
                  }
                }
                n517 = Array Subset(array=w915, index="拟合起点", length=w916) -> (w918:dbl[])
                n518 = Bundle("波长范围"=w913, "Filtered X"=w915) -> (w914:cluster{"波长范围 ":dbl[], "Filtered X":dbl[]})  [unwired: 1 in]
                n519 = case shown="真" "是否拟合" {
                  tunnel: w918 -> [w951 w957]
                  tunnel: w919 -> [_ w956]
                  tunnel: [w951 w955] -> w933
                  tunnel: w914 -> [_ w953]
                  frame False {
                  }
                  frame True {
                    n520 = call "转换至动态数据7"("Array"=w957) -> ("Dynamic Data Type"=w962:dynamicdata)  [unwired: 3 in]
                    n521 = call "转换至动态数据8"("Array"=w956) -> ("Dynamic Data Type"=w963:dynamicdata)  [unwired: 3 in]
                    n522 = call "曲线拟合2"("Locations"=w963, "Signals"=w962) -> ("best fit"=w960:dynamicdata, "non-linear coefficients"=w961:dynamicdata)  [unwired: 5 in, 3 out]
                    n523 = call "从动态数据转换3"("Dynamic Data Type"=w961) -> ("Array"=w964:dbl[])  [unwired: 3 in]
                    n524 = call "从动态数据转换4"("Dynamic Data Type"=w960) -> ("Array"=w955:dbl[])  [unwired: 3 in]
                    n525 = Index Array(array=w964, index #1=0 ("索引"), index #2=1 ("索引")) -> (element #1=w966:dbl, element #2=w965:dbl)
                    n526 = local write "拟合参数"(w964) -> ()
                    n527 = local write "xc"(w966) -> ()
                    n528 = Bundle(w956, "Array"=w955) -> (w954:cluster{dbl[], "Array":dbl[]})  [unwired: 1 in]
                    n529 = local write "w"(w965) -> ()
                    n530 = Build Array(w953, w954) -> (→"best fit":cluster{"波长范围 ":dbl[], "Array":dbl[]}[])
                  }
                }
                n531 = Build Array(w919, w922, w933, w912) -> (w921:dbl[][])
              }
              frame #4 {
                n532 = case shown="真" "是否保存" {
                  tunnel: w988 -> [_ w992]
                  frame False {
                  }
                  frame True {
                    n533 = Get Date/Time In Seconds() -> (seconds since 1Jan1904=w1006:timestamp)
                    n534 = Get Date/Time String(date format (0)=enum16{"short", "long", "abbreviated"}."abbreviated" ("日期格式(0)"), seconds (now)=w1006, want seconds? (F)=TRUE ("需要秒？(F)")) -> (date string=w1004:string, time string=w1005:string)
                    n535 = Search and Replace String(replace all?=TRUE ("替换全部？(F)"), input string=w1005, search string=":" ("搜索字符串"), replace string="-" ("替换字符串(\"\")")) -> (result string=w1003:string)  [unwired: 4 in, 3 out]
                    n536 = local read "最终存储路径 2"() -> (w1007:path)
                    n537 = Path To String(path=w1007) -> (string=w1010:string)
                    n538 = Concatenate Strings(w1010, w1004, w1003, "光谱" ("字符串"), ".xls" ("字符串")) -> (w1009:string)
                    n539 = String To Path(string=w1009) -> (path=w1008:path)
                    n540 = call-poly <vilib>:"Write Delimited Spreadsheet.vi"("file path (dialog if empty)"=w1008, "format (%.3f)"="%.16f", "2D data"=w992, "append to file? (new file:F)"=TRUE ("append to file? (F)"), "transpose? (no:F)"=TRUE ("transpose? (F)")) -> ()  [unwired: 9 in, 2 out]
                  }
                }
                n541 = case shown="真" "Save Backlight" {
                  frame False {
                  }
                  frame True {
                    w1011 = TRUE ("删除背景光")
                    n542 = local read "Data"() -> (w1013:i32[][])
                    n543 = local write "Backlight"(w1013) -> ()
                    n544 = local write "cut backlight"(w1011) -> ()
                    n545 = local write "backlight"(w1011) -> ()
                    n546 = local write "Save Backlight"(FALSE ("Save Backlight")) -> ()
                  }
                }
                n547 = local write "CCD Busy"(FALSE ("CCD Busy")) -> ()
              }
            }
          }
        }
        n548 = case shown="假" "Setup" {
          tunnel: w848 -> [_ w1027]
          tunnel: w849 -> [_ w1026]
          frame False {
          }
          frame True {
            n549 = stacked-sequence {
              tunnel: w1027 -> [_ w1041 _]
              tunnel: w1026 -> [_ w1029 _]
              frame #0 {
                n550 = local write "indicator"("Setting up the detector" ("indicator")) -> ()
              }
              frame #1 {
                w1039 = 1 items=["JYMCD_ACQ_FORMAT_IMAGE", "JYMCD_ACQ_FORMAT_SCAN"] ("Acquisition type")
                n551 = local read "Gain Number"() -> (w1034:i32[])
                n552 = local read "GAIN"() -> (w1030:u16)
                n553 = local read "ADC Number"() -> (w1035:i32[])
                n554 = local read "ADC"() -> (w1031:u16)
                n555 = Index Array(array=w1034, index=w1030) -> (element=w1032:i32)
                n556 = Index Array(array=w1035, index=w1031) -> (element=w1033:i32)
                n557 = local read "Number of Areas :"() -> (w1037:u16)
                n558 = local read "areas :"() -> (w1038:i32[][])
                n559 = call "Setup CCD.vi"("numAreas"=w1037, "areas :"=w1038, "JYCCDLib.IJYCCDReqd"=w1029, "entrée d'erreur (pas d'erreur)"=w1041, "Acquisition type"=w1039, "Gain"=w1032, "Select ADC"=w1033, "Integration time(ms)"="Integration time (ms) :") -> ("DataSize"=→"DataSize":i32)  [unwired: 1 out]
                "JYCCDLib.IJYCCDReqd" <- w1029
              }
              frame #2 {
                w1042 = TRUE ("Visible")
                n560 = property on="Continuous" class="Bool (严格)"("Visible"=w1042) -> ()  [unwired: 2 in, 2 out]
                n561 = property on="Acquire" class="Bool"("Visible"=w1042) -> ()  [unwired: 2 in, 2 out]
                n562 = local write "indicator"("Ready !" ("indicator")) -> ()
              }
            }
          }
        }
        n563 = case shown="假" "Temperature" {
          tunnel: w849 -> [_ w1016]
          tunnel: w848 -> [_ w1015]
          frame False {
            n564 = property on="temp graph" class="WFChart (严格)"("Visible"=FALSE) -> ()  [unwired: 2 in, 2 out]
          }
          frame True {
            n565 = stacked-sequence {
              tunnel: w1016 -> [_ w1021]
              tunnel: w1015 -> [_ w1020]
              frame #0 {
                n566 = property on="temp graph" class="WFChart (严格)"("Visible"=TRUE) -> ()  [unwired: 2 in, 2 out]
              }
              frame #1 {
                w1019 = u16 0 items=["° Celsius", "Kelvin", "° Farenheit"] ("units")
                n567 = call "read temperature.vi"("entrée d'erreur (pas d'erreur)"=w1020, "units"=w1019, "JYCCDLib.IJYCCDReqd"=w1021) -> ("Current Temperature"=w1018:dbl)
                n568 = local write "temp graph"(w1018) -> ()
              }
            }
          }
        }
        n569 = Wait Until Next ms Multiple(millisecond multiple=u32 50 ("n millisecondes")) -> ()  [unwired: 1 out]
      }
    }
    frame #7 {
      n570 = Close Reference(reference=w1045, error in (no error)=w1044) -> ()  [unwired: 1 out]
    }
  }
  n571 = stacked-sequence {
    seq-local: [_ _ w1055 _ _] -> [_ _ _ w1065 w1070]
    seq-local: [_ _ w1054 _ _] -> [_ _ _ w1064 _]
    seq-local: [_ _ _ w1063 _] -> [_ _ _ _ _]
    frame #0 {
      n572 = call "Get Monos From Config Browser.vi"() -> ("UniqueIDs"=w1050:string[], "Mono ID"=w1051:string[])  [unwired: 3 in, 1 out]
      n573 = Build Cluster Array(w1051, w1050) -> (w1048:cluster{"String":string, "String":string}[])
      n574 = property on="Mono ID" class="CmbBox"("Strings And Values []"=w1048) -> ()  [unwired: 2 in, 2 out]
      n575 = Index Array(array=w1048, index=0) -> (element=w1049:cluster{"String":string, "String":string})
      n576 = Unbundle(w1049) -> ("String"=w1046:string)  [unwired: 1 out]
      "Current UniqueID" <- w1046
      n577 = local write "Mono ID"(w1046) -> ()
    }
    frame #1 {
      n578 = while {
        stop <- "Connect" stop-if-true
        n579 = local read "Mono ID"() -> (w1052:string)
        n580 = local write "Current UniqueID"(w1052) -> ()
      }
    }
    frame #2 {
      n581 = local read "Mono ID"() -> (w1057:string)
      n582 = call "JYInitMono.vi"("Unique ID"=w1057, "Force Init"="Force\nInitialization") -> ("Refnum out"=w1055:refnum<k7>, "Initialized"=→"Initialized JY":bool, "error out"=w1054:errorcluster)  [unwired: 9 in, 2 out]
    }
    frame #3 {
      n583 = call "Show Current Grating.vi"("Refnum in"=w1065, "error in (no error)"=w1064) -> ("Gratings"=w1066:dbl[], "Grating Index"=w1060:i32, "Current Grating"=w1062:dbl, "Current Description"=w1059:string, "error out"=w1063:errorcluster)  [unwired: 5 in, 4 out]
      "Gratings" <- w1066
      n584 = local write "Current Grating"(w1062) -> ()
      n585 = local write "Current Description"(w1059) -> ()
      n586 = Number To Decimal String(number=w1066) -> (decimal integer string=w1068:string[])  [unwired: 1 in]
      n587 = Number To Decimal String(number=w1060) -> (decimal integer string=w1061:string)  [unwired: 1 in]
      n588 = property on="Target Grating" class="CmbBox"("Value"=w1061) -> ()  [unwired: 2 in, 2 out]
      n589 = Build Cluster Array(w1068, string[] ["1", "2", "3"]) -> (w1069:cluster{"Numeric":string, string}[])
      n590 = property on="Target Grating" class="CmbBox"("Strings And Values []"=w1069) -> ()  [unwired: 2 in, 2 out]
    }
    frame #4 {
      n591 = while {
        tunnel: w1070 -> [w1072]
        stop <- w1071 stop-if-true
        n592 = stacked-sequence {
          seq-local: [w1076 _ _ _ _] -> [_ w1083 w1094 _ w1102]
          seq-local: [w1075 _ _ _ _] -> [_ w1082 w1093 _ _]
          seq-local: [_ w1081 _ _ _] -> [_ _ _ _ _]
          seq-local: [_ w1080 _ _ _] -> [_ _ _ _ _]
          seq-local: [_ _ w1086 _ _] -> [_ _ _ _ _]
          seq-local: [_ _ w1085 _ _] -> [_ _ _ w1096 _]
          tunnel: w1072 -> [w1074 _ _ w1097 _]
          frame #0 {
            n593 = call "Show Current Grating.vi"("Refnum in"=w1074) -> ("Grating Index"=→"Grating Index":i32, "Current Grating"=→"Current Grating":dbl, "Current Description"=→"Current Description":string, "error out"=w1075:errorcluster, "JYMONOLib.IJYMonoReqd"=w1076:refnum<k7>)  [unwired: 6 in, 4 out]
          }
          frame #1 {
            n594 = call "JYGetCurrentWL.vi"("error in (no error)"=w1082, "JYMONOLib.IJYMonoReqd"=w1083) -> ("error out"=w1080:errorcluster, "Units"=→"Units":string, "Current WL"=→"Current WL":dbl, "JYMONOLib.IJYMonoReqd 2"=w1081:refnum<k7>)  [unwired: 6 in]
          }
          frame #2 {
            w1091 = u16 1 items=["Entrance", "Exit"] ("Mirror Number")
            w1092 = u16 0 items=["Entrance", "Exit"] ("Mirror Number")
            n595 = call "JYGetMirrorPos.vi"("error in (no error)"=w1093, "Mirror"=w1092, "Refnum In"=w1094) -> ("error out"=w1089:errorcluster, "Current Mirror Position"=→"Entrance Mirror\nPosition":i32, "Refnum Out"=w1090:refnum<k7>)  [unwired: 1 in]
            n596 = call "JYGetMirrorPos.vi"("error in (no error)"=w1089, "Mirror"=w1091, "Refnum In"=w1090) -> ("error out"=w1085:errorcluster, "Current Mirror Position"=→"Exit Mirror\nPosition":i32, "Refnum Out"=w1086:refnum<k7>)  [unwired: 1 in]
          }
          frame #3 {
            w1099 = u16 0 items=["Front Entrance", "Side Entrance", "Front Exit", "Side Exit", "First Intermediate", "Second Intermediate"] ("Slit")
            n597 = call "JYGetSlits.vi"("MonoRefNum IN"=w1097, "Slit"=w1099, "error in (no error)"=w1096) -> ("Units"=→"Units 2":string, "Slit Width"=→"Front Entrance":dbl, "error out"=→"error out":errorcluster)  [unwired: 13 in, 1 out]
          }
          frame #4 {
            n598 = case shown="假" "Move To\nTarget Positions" {
              tunnel: w1102 -> [_ w1103]
              frame False {
              }
              frame True {
                n599 = stacked-sequence {
                  seq-local: [w1105 _ _ _] -> [_ w1111 _ _]
                  seq-local: [_ w1109 _ _] -> [_ _ w1126 _]
                  seq-local: [_ _ w1113 _] -> [_ _ _ w1132]
                  seq-local: [_ _ _ w1129] -> [_ _ _ _]
                  tunnel: w1103 -> [w1107 w1110 w1124 w1133]
                  frame #0 {
                    n600 = property on="Target Grating" class="CmbBox"() -> ("Value"=w1104:string)  [unwired: 2 in, 2 out]
                    n601 = local read "error out"() -> (w1106:errorcluster)
                    n602 = Decimal String To Number(string=w1104) -> (number=w1108:i32)  [unwired: 2 in, 1 out]
                    n603 = call "JYTurret.vi"("error in (no error)"=w1106, "Grating Index"=w1108, "JYMONOLib.IJYMonoReqd"=w1107) -> ("error out"=w1105:errorcluster)  [unwired: 2 out]
                  }
                  frame #1 {
                    # "Move Grating to Target Position"
                    n604 = call "JYMoveToWavelength.vi"("error in (no error)"=w1111, "Target WL"="Target WL", "RefNum In"=w1110) -> ("error out"=w1109:errorcluster)  [unwired: 1 in, 2 out]
                  }
                  frame #2 {
                    w1119 = u16 1 items=["Entrance", "Exit"] ("Mirror Number")
                    w1118 = u16 0 items=["Entrance", "Exit"] ("Mirror Number")
                    w1125 = u16 1 items=["Entrance", "Exit", "Front", "Side"] ("Mirror Number")
                    w1128 = u16 0 items=["Entrance", "Exit", "Front", "Side"] ("Mirror Number")
                    # "Move Mirrors"
                    n605 = call "JYMirrorMove.vi"("error in (no error)"=w1126, "Mirror Position"="Entrance Mirror", "Mirror Number"=w1128, "RefNum In"=w1124) -> ("error out"=w1123:errorcluster)  [unwired: 6 in, 1 out]
                    n606 = call "JYMirrorMove.vi"("error in (no error)"=w1123, "Mirror Position"="Exit Mirror", "Mirror Number"=w1125, "RefNum In"=w1124) -> ("error out"=w1116:errorcluster, "MonoRefNum Out"=w1117:refnum<k7>)  [unwired: 6 in]
                    n607 = call "JYGetMirrorPos.vi"("error in (no error)"=w1116, "Mirror"=w1118, "Refnum In"=w1117) -> ("error out"=w1121:errorcluster, "Current Mirror Position"=w1115:i32, "Refnum Out"=w1120:refnum<k7>)  [unwired: 1 in]
                    n608 = local write "Entrance Mirror\nPosition"(w1115) -> ()
                    n609 = call "JYGetMirrorPos.vi"("error in (no error)"=w1121, "Mirror"=w1119, "Refnum In"=w1120) -> ("error out"=w1113:errorcluster, "Current Mirror Position"=w1114:i32)  [unwired: 1 in, 1 out]
                    n610 = local write "Exit Mirror\nPosition"(w1114) -> ()
                  }
                  frame #3 {
                    w1131 = u16 0 items=["Front Entrance", "Side Entrance", "Front Exit", "Side Exit", "First Intermediate", "Second Intermediate"] ("Slit")
                    # "Set New Slit Positions"
                    n611 = call "JYSlits.vi"("JYMONOLib.IJYMonoReqd"=w1133, "Slit"=w1131, "error in (no error)"=w1132, "Slit Width"="Target\nFront Entrance") -> ("error out"=w1129:errorcluster)  [unwired: 1 in, 1 out]
                  }
                }
              }
            }
          }
        }
        n612 = local read "Close"() -> (w1071:bool)
      }
    }
  }
  n613 = flat-sequence {
    frame #0 {
      n614 = call <vilib>:"Create Report.vi"("window state (normal)"=T3."no change", "report type"=Report_Type."Excel", "template (empty)"=path "D:/desktop/train/TEST1/Save/516中心波长.xlsx") -> ("report out"=w1140:refnum<class "NI_report.lvclass">, "error out"=w1139:errorcluster)  [unwired: 11 in]
      n615 = call-poly <vilib>:"Excel Get Data.vi"("report in"=w1140, "data type"=string[][] [], "error in (no error)"=w1139) -> ("report out"=w1135:refnum<class "NI_report.lvclass">, "data"=w1143:string[][], "error out"=w1134:errorcluster)  [unwired: 10 in]
      n616 = call-dynamic "Dispose Report.vi"("report in"=w1135, "error in (no error)"=w1134) -> ()  [unwired: 13 in, 1 out]
      n617 = Index Array(array=w1143, index (col)=0 ("禁用的索引 (列)")) -> (element=w1145:string[])  [unwired: 1 in]
      n618 = Fract/Exp String To Number(string=w1145) -> (number=→"波长范围":dbl[])  [unwired: 3 in, 1 out]
    }
  }
